vi "FL30XX.VI"() -> ()   [LabVIEW 2015]
uses:
  board.vis/Globals.vi
  board.vis/ESLSCDLL.lvlib
  board.vis/ESLSCDLL.dll
panel:
  in  "abort":bool
  in  "FFT mode":T1(ring)
  in  "is FFT":bool
  out "ADSC value":u32
  in  "Read ADSC":bool
  in  "Reset DSC":bool
  in  "CC trigger":enum32{"XCK", "Ext. Trig.", "DAT"}(ring)
  in  "STSlope":enum32{"pos", "neg", "both"}(ring)
  in  "BTSlope":enum32{"neg", "pos", "both"}(ring)=enum."pos"
  in  "btime[ms]":dbl=30.0 format="%.3f"
  out "Block on":bool
  out "String":string="with int trig:\nset exp.time accordingly\ncheck with scope!"
  in  "STI":T2(ring)=enum."STimer"
  out "TDC 2":u16
  out "TDC 1":u16
  in  "startevent":bool
  in  "BTI":enum32{"I", "S1", "S2", "S1&S2", "BTimer"}(ring)=enum."BTimer"
  in  "shutter open":bool
  in  "value black":u32
  in  "value white":u32=65535
  in  "show greyscale viewer":bool
  out "mean 3":dbl=-1.0 format="%0#.1f"
  out "tRMS 3":dbl=-1.0 format="%0#.1f"
  out "meanB":dbl=7869.371428571429 format="%0#.1f"
  out "tRMSB":dbl=13.410972192676741 format="%0#.1f"
  in  "Pixel for Graph":u32(slide)=660 max=3000 scale=0.0..1087.0
  in  "fast test\ncontinuous":bool
  out "One Pixel Graph":u16[][](graph)=[[50944, 37299, 23643, 29270, 42944, 50969, 37301, 23634, 29310, 42916, 50937, 37273, 23614, 29274, 42951, 50937, 37273, 23623, 29272, 42950, 50962, 37247, 23599, 29236, 42962, 50936, 37300, 23595, 29263, 42929, 50960, 37290, 23598, 29279, 42957, 50913, 37317, 23578, 29305, 42929, 50968, 37259, 23609, 29292, 42945, 50893, 37300, 23589, 29261, 42955, 50920, 37282, 23639, 29263, 42945, 50934, 37283, 23614, 29291, 42918, 50913, 37257, 23579, 29291, 42942, 50959, 37282, 23546, 29281, 42947, 50936, 37291, 23618, 29269, 42975, 50886, 37275, 23582, 29349, 42945, 50916, 37241, 23621, 29295, 42960, 50911, 37268, 23591, 29293, 42935, 50920, 37282, 23580, 29297, 42905, 50935, 37262, 23651, 29293, 42972, 50942, 37321, 23596, 29274, 42941, 50931, 37251, 23635, 29286, 42978, 50922, 37296, 23575, 29289, 42930, 50937, 37245, 23622, 29273, 42966, 50915, 37257, 23583, 29291, 42935, 50904, 37260, 23580, 29276, 42947, 50900, 37261, 23616, 29273, 42934, 50894, 37296, 23594, 29275, 42946, 50925, 37263, 23603, 29280, 42945, 50895, 37270, 23607, 29241, 42924, 50945, 37219, 23609, 29283, 42998, 50911, 37270, 23580, 29303, 42949, 50939, 37239, 23605, 29279, 42957, 50863, 37246, 23602, 29277, 42954, 50928, 37235, 23581, 29261, 42938, 50910, 37257, 23587, 29290, 42968, 50905, 37279, 23586, 29318, 42951, 50927, 37227, 23626, 29313, 42937, 50930, 37271, 23565, 29310, 42931, 50951, 37220, 23620, 29305, 42975, 50892, 37264, 23585, 29313, 42946, 50912, 37261, 23591, 29299, 42971, 50927, 37277, 23588, 29310, 42990, 50910, 37298, 23578, 29255, 42956, 50941, 37289, 23612, 29292, 43046, 50897, 37282, 23581, 29298, 42948, 50916, 37252, 23580, 29299, 42965, 50871, 37256, 23615, 29311, 42989, 50917, 37242, 23567, 29328, 42923, 50952, 37220, 23614, 29299, 42967, 50884, 37266, 23556, 29324, 42964, 50907, 37242, 23562, 29316, 42960, 50848, 37260, 23579, 29285, 42986, 50925, 37229, 23582, 29300, 42956, 50898, 37261, 23588, 29283, 42965, 50909, 37242, 23548, 29313, 42953, 50928, 37266, 23599, 29269, 42951, 50901, 37275, 23577, 29292, 42966, 50882, 37256, 23572, 29293, 42933, 50878, 37265, 23599, 29326, 42990, 50908, 37285, 23534, 29333, 42937, 50875, 37251, 23590, 29313, 43002, 50920, 37258, 23588, 29337, 42975, 50941, 37239, 23560, 29306, 42969, 50883, 37244, 23567, 29315, 42951, 50905, 37262, 23579, 29339, 42995, 50936, 37240, 23593, 29321, 43034, 50890, 37262, 23533, 29333, 42993, 50929, 37210, 23580, 29291, 42992, 50871, 37260, 23574, 29346, 42991, 50901, 37242, 23586, 29358, 42953, 50895, 37237, 23586, 29303, 43004, 50899, 37252, 23538, 29332, 42954, 50907, 37243, 23587, 29302, 43013, 50874, 37240, 23579, 29306, 42979, 50883, 37242, 23598, 29300, 42969, 50933, 37241, 23571, 29298, 42988, 50863, 37276, 23525, 29321, 42994, 50882, 37228, 23551, 29299, 42981, 50878, 37206, 23545, 29367, 42987, 50915, 37225, 23550, 29315, 42985, 50896, 37239, 23533, 29336, 42985, 50904, 37237, 23525, 29331, 42976, 50905, 37232, 23569, 29341, 42978, 50875, 37229, 23558, 29320, 42971, 50874, 37226, 23576, 29327, 43000, 50940, 37258, 23550, 29339, 43011, 50910, 37226, 23567, 29312, 42975, 50885, 37233, 23535, 29350, 42984, 50876, 37205, 23532, 29335, 42948, 50887, 37214, 23575, 29328, 42984, 50894, 37236, 23563, 29365, 42996, 50944, 37248, 23572, 29326, 43012, 50893, 37236, 23573, 29340, 43019, 50883, 37199, 23530, 29375, 42995, 50914, 37201, 23608, 29323, 43008, 50883, 37216, 23552, 29381, 42977, 50894, 37240, 23572, 29367, 43030, 50880, 37205, 23586, 29302, 43016, 50874, 37238, 23561, 29326, 43000]]
  in  "refresh":bool
  out "C 8":bool
  out "C 7":bool
  out "C 6":bool
  out "C 5":bool
  out "C 4":bool
  out "C 3":bool
  out "C 2":bool
  out "(LastCAM) \n        C1":bool
  out "cool_temp Reg":u32 format="%032b"
  in  "cool":u8 caption="(0 to 7)"
  in  "Offset":bool
  out "Signal Cam 4":u16[](graph)
  out "Signal Cam 3":u16[](graph)
  out "mean 2":dbl=-1.0 format="%0#.1f"
  out "meanA":dbl=33883.361224489796 format="%0#.1f"
  in  "TRMS Pix":u32=550 max=1087
  out "tRMS 2":dbl=-1.0 format="%0#.1f"
  in  "Board select":string(combo)
  in  "Initialize":bool
  in  "About S0":bool
  in  "send all":bool
  in  "DAC 8/ 1":u16=54400
  in  "DAC 3/ 1":u16=54540
  in  "DAC 7/ 1":u16=54670
  in  "DAC 2/ 1":u16=54600
  in  "DAC 6/ 1":u16=54880
  in  "DAC 1/ 1":u16=54530
  in  "DAC 5/ 1":u16=54600
  in  "DAC 4/ 1":u16=54590
  in  "custom patt: 14bits pattern hex (14bit)":u16=100 format="%x"
  out "pattern dec":fxp<+,14,14>
  in  "ADC mode":enum32{"1", "2", "3"}(radio)=enum."3"
  out "Signal Cam 2":u16[](graph)
  out "tRMSA":dbl=19568.501745308375 format="%0#.1f"
  in  "Gain":bool
  in  "framewise\ncontinuous":bool
  out "curr_read_block":u8=1
  out "Measure on":bool
  in  "no.of blocks (nob)":u32=1 min=1
  in  "block":u32(slide)=1 min=1 max=1 scale=0.9..1.0
  out "Signal Board 2 / Cam1":u16[](graph)
  out "Signal Board 1 / Cam1":u16[](graph)=[65412, 65216, 0, 1, 0, 151, 0, 0, 0, 0, 50811, 50676, 50513, 50360, 50171, 49982, 49793, 49614, 49450, 49306, 49194, 48996, 48865, 48698, 48506, 48325, 48153, 47990, 47816, 47655, 47545, 47383, 47176, 47044, 46862, 46698, 46512, 46359, 46209, 46025, 45899, 45678, 45593, 45374, 45201, 45026, 44901, 44695, 44537, 44379, 44241, 44106, 43900, 43719, 43563, 43392, 43207, 43077, 42921, 42783, 42619, 42451, 42281, 42085, 41924, 41737, 41582, 41431, 41307, 41149, 40966, 40770, 40597, 40456, 40278, 40139, 39968, 39845, 39651, 39489, 39284, 39124, 38971, 38800, 38643, 38498, 38339, 38180, 38005, 37872, 37703, 37496, 37324, 37175, 37020, 36894, 36678, 36546, 36347, 36213, 36015, 35858, 35661, 35544, 35350, 35216, 35068, 34907, 34746, 34570, 34372, 34178, 34055, 33869, 33726, 33574, 33440, 33278, 33068, 32945, 32751, 32561, 32423, 32272, 32099, 31954, 31774, 31588, 31409, 31263, 31150, 30968, 30786, 30618, 30484, 30305, 30154, 29940, 29781, 29638, 29458, 29323, 29146, 28997, 28856, 28632, 28514, 28322, 28173, 28003, 27866, 27660, 27524, 27315, 27163, 27002, 26861, 26661, 26542, 26378, 26190, 26055, 25854, 25683, 25541, 25367, 25203, 25023, 24875, 24711, 24556, 24366, 24240, 24050, 23898, 23731, 23569, 23409, 23279, 23087, 22906, 22730, 22578, 22400, 22255, 22097, 21944, 21800, 21577, 21428, 21245, 21125, 20911, 20770, 20619, 20443, 20311, 20126, 19980, 19760, 19614, 19449, 19316, 19119, 18986, 18852, 18640, 18509, 18296, 18156, 17941, 17807, 17613, 17534, 17339, 17189, 17022, 16864, 16682, 16488, 16314, 16172, 15994, 15868, 15693, 15575, 15402, 15216, 15026, 14844, 14675, 14496, 14324, 14245, 14076, 13910, 13712, 13577, 13385, 13228, 12999, 12884, 12730, 12579, 12441, 12264, 12086, 11953, 11730, 11532, 11400, 11227, 11053, 10936, 10748, 10627, 10422, 10270, 10085, 9907, 9785, 9589, 9456, 9249, 9109, 8925, 8763, 8588, 8460, 8287, 8117, 7943, 7815, 7654, 7440, 7297, 7135, 6957, 6789, 6631, 6490, 6301, 6139, 5965, 5813, 5661, 5492, 5342, 5212, 4985, 4872, 4637, 4441, 4306, 4206, 4013, 3889, 3690, 3542, 3385, 3189, 3025, 2874, 2709, 2513, 2368, 2205, 2056, 1910, 1719, 1555, 1402, 1212, 1082, 907, 752, 605, 445, 258, 72, 0, 0, 0, 0, 0, 0, 0, 0, 0, 0, 0, 0, 151, 312, 511, 714, 849, 1024, 1166, 1300, 1482, 1649, 1819, 2010, 2112, 2346, 2468, 2649, 2803, 2967, 3134, 3309, 3503, 3626, 3822, 3902, 4115, 4247, 4442, 4599, 4750, 4965, 5102, 5270, 5376, 5612, 5729, 5904, 6071, 6270, 6459, 6598, 6780, 6883, 7065, 7226, 7356, 7543, 7760, 7915, 8075, 8235, 8382, 8518, 8701, 8868, 9028, 9228, 9389, 9560, 9740, 9861, 10039, 10193, 10345, 10490, 10703, 10875, 11058, 11215, 11376, 11527, 11658, 11832, 11992, 12171, 12336, 12545, 12706, 12875, 13023, 13161, 13315, 13483, 13636, 13778, 14006, 14173, 14347, 14464, 14689, 14809, 14997, 15163, 15301, 15499, 15644, 15844, 15961, 16116, 16283, 16443, 16623, 16806, 16971, 17146, 17333, 17437, 17646, 17763, 17935, 18076, 18241, 18408, 18591, 18758, 18897, 19096, 19258, 19440, 19564, 19754, 19895, 20074, 20212, 20376, 20542, 20753, 20884, 21097, 21209, 21412, 21546, 21692, 21879, 22022, 22223, 22345, 22551, 22715, 22894, 23017, 23193, 23325, 23485, 23694, 23841, 23987, 24201, 24357, 24522, 24691, 24825, 24954, 25106, 25283, 25468, 25683, 25862, 26023, 26162, 26287, 26450, 26604, 26776, 26941, 27150, 27306, 27475, 27649, 27799, 27935, 28099, 28219, 28422, 28589, 28811, 28965, 29145, 29250, 29438, 29573, 29718, 29898, 30077, 30229, 30440, 30612, 30759, 30921, 31056, 31211, 31363, 31533, 31712, 31879, 32067, 32239, 32414, 32534, 32696, 32850, 33030, 33204, 33360, 33537, 33724, 33842, 34021, 34178, 34329, 34488, 34642, 34835, 35007, 35191, 35336, 35497, 35663, 35816, 35973, 36131, 36313, 36476, 36625, 36803, 36950, 37174, 37281, 37426, 37646, 37801, 37959, 38128, 38270, 38460, 38603, 38746, 38931, 39098, 39240, 39453, 39608, 39758, 39913, 40107, 40240, 40411, 40603, 40736, 40910, 41078, 41218, 41421, 41540, 41722, 41844, 42060, 42227, 42437, 42539, 42747, 42860, 43039, 43169, 43356, 43493, 43688, 43818, 44024, 44220, 44357, 44504, 44666, 44818, 44990, 45166, 45331, 45498, 45656, 45806, 45964, 46151, 46312, 46469, 46655, 46820, 46956, 47139, 47276, 47489, 47620, 47774, 47975, 48121, 48294, 48468, 48599, 48782, 48923, 49091, 49240, 49408, 49596, 49777, 49943, 50096, 50263, 50415, 50577, 50740, 50910, 51082, 51247, 51421, 51570, 51778, 51885, 52034, 52181, 52353, 52531, 52735, 52898, 53058, 53223, 53371, 53516, 53666, 53826, 54005, 54205, 54349, 54512, 54736, 54859, 55012, 55161, 55342, 55492, 55645, 55844, 56018, 56186, 56352, 56502, 56656, 56808, 56958, 57179, 57337, 57518, 57656, 57795, 57962, 58123, 58277, 58458, 58625, 58804, 58966, 59150, 59290, 59459, 59580, 59791, 59941, 60088, 60291, 60460, 60650, 60812, 60923, 61089, 61240, 61405, 61541, 61790, 61941, 62115, 62312, 62444, 62600, 62748, 62871, 63033, 63232, 63414, 63536, 63763, 63880, 64071, 64261, 64380, 64539, 64683, 64825, 65040, 65200, 65394, 65535, 65535, 65535, 65535, 65535, 65535, 65535, 65535, 65535, 65535, 65535, 65535, 65535, 65535, 65535, 65535, 65535, 65535, 65535, 65535, 65535, 65535, 65535, 65535, 65524, 65296, 65146, 64951, 64825, 64641, 64532, 64393, 64226, 64044, 63834, 63698, 63474, 63328, 63164, 63032, 62887, 62732, 62570, 62386, 62221, 62017, 61833, 61682, 61546, 61383, 61215, 61054, 60948, 60729, 60571, 60359, 60199, 60035, 59886, 59745, 59581, 59449, 59265, 59104, 58921, 58730, 58519, 58380, 58244, 58091, 57962, 57834, 57638, 57364, 57279, 57079, 56920, 56742, 56603, 56469, 56296, 56154, 55934, 55788, 55584, 55418, 55262, 55114, 54960, 54795, 54678, 54443, 54307, 54139, 53955, 53792, 53623, 53469, 53299, 53172, 53022, 52830, 52666, 52490, 52310, 52166, 51986, 51857, 51662, 51548, 51342, 51181, 51000, 50837, 50660, 50492, 50391, 50188, 50085, 49874, 49714, 49544, 49353, 49160, 49039, 48877, 48737, 48557, 48401, 48225, 48041, 47935, 47725, 47585, 47401, 47231, 47125, 46913, 46782, 46573, 46416, 46223, 46071, 45886, 45758, 45614, 45445, 45276, 45122, 44964, 44782, 44608, 44424, 44220, 44103, 43949, 43789, 43649, 43479, 43305, 43148, 42969, 42834, 42621, 42507, 42316, 42140, 41985, 41838, 41659, 41486, 41342, 41163, 41025, 40849, 40651, 40502, 40364, 40171, 40025, 39852, 39696, 39497, 39388, 39188, 39029, 38880, 38701, 38568, 38414, 38214, 38081, 37855, 37727, 37486, 37388, 37210, 37080, 36908, 36768, 36606, 36395, 36247, 36093, 35904, 35738, 35582, 35420, 35274, 35111, 34923, 34765, 34602, 34448, 34314, 34120, 33941, 33814, 33596, 33493, 33276, 33132, 32966, 32821, 32630, 32501, 32322, 32144, 31968, 31816, 31667, 31515, 31347, 31183, 31019, 30860, 30678, 30521, 30333, 30179, 30001, 29870, 29707, 29566, 29413, 29221, 29032, 28817, 28696, 28474, 28364, 28217, 28054, 27918, 27741, 27575, 27401, 27211, 27035, 26852, 26699, 26562, 26404, 26274, 26125, 25942, 25754, 25563, 25405, 25223, 25082, 24938, 24794, 24628, 24465, 24277, 24152, 23901, 23772, 23583, 23462, 23288, 23165, 22985, 22829, 22650, 22457, 22302, 22085, 21979, 21818, 21652, 21537, 21331, 21172, 20948, 20846, 20664, 20477, 20358, 20181, 20033, 19847, 19702, 19524, 19360, 19171, 19025, 18836, 18707, 18533, 18375, 18219, 18066, 17894, 17716, 17586, 17348, 17195, 17043, 16880, 16746, 16540, 16414, 16226, 16086, 15916, 15761, 15567, 15436, 15228, 15083, 14916, 14783, 14582, 14447, 14259, 14103, 13948, 13777, 13612, 13443, 13285, 13106, 12993, 12807, 12591, 12454, 12268, 12125, 11948, 11817, 65534, 65535, 0, 0, 2, 0]
  out "# boards \ndetected":u32=1
  in  "alloc mem":bool
  out "FREE \nRAM MB":dbl=29213.2109375
  out "BUILT-IN\nRAM MB":dbl=32640.29296875
  out "SEC":dbl=0.1
  out "MB RAM":dbl=1.03759765625
  in  "SDAT in 10ns":u32
  in  "exit":bool
  in  "start":bool
  in  "sample":u32(slide)=151 min=1 max=20 scale=1.0..20.0
  in  "no.of samples (nos)":u32=20 min=2
  in  "stime[ms]":dbl=1.0 format="%.3f"
  # "press \"Initialize\", then \"alloc mem\"\nand then \"start\""
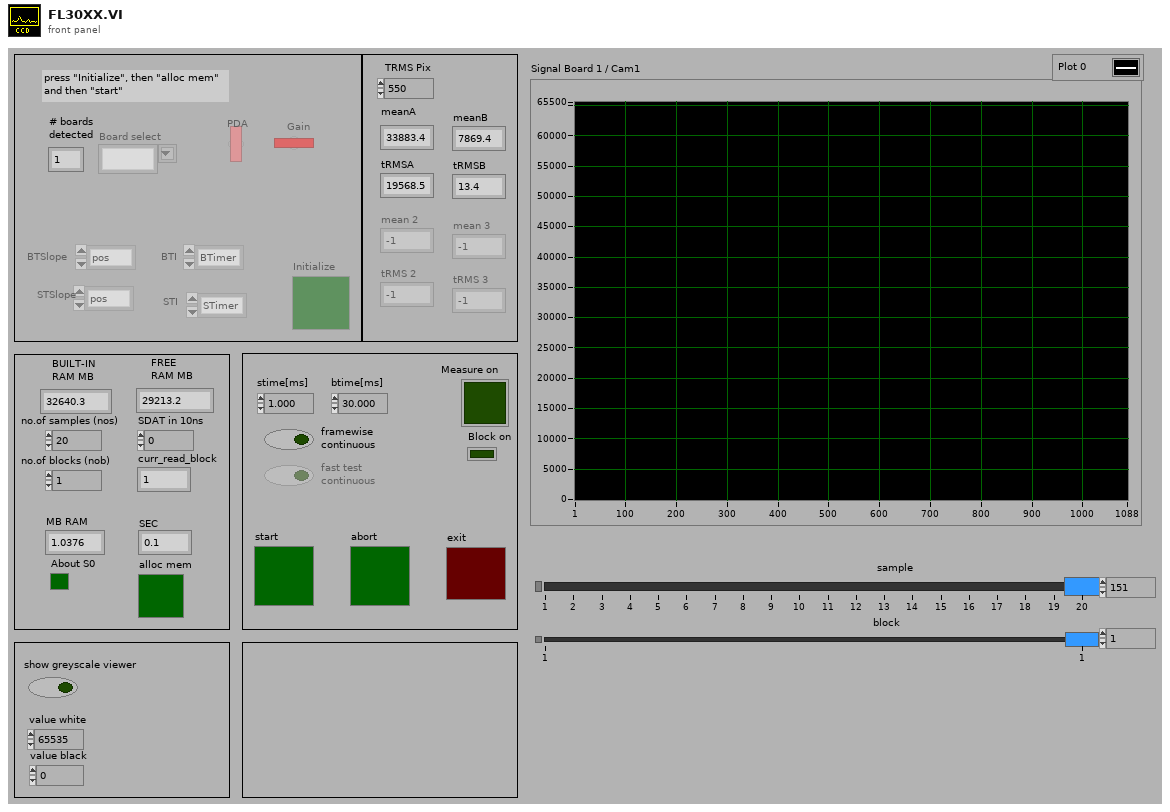
[diagram p1: front panel]
types:
  T1 = enum32{"Full Binning", "Region of Interest", "Area"}
  T2 = enum32{"I", "S1", "S2", "unused", "STimer", "ASL"}
  T3 = enum32{"XCK", "Reg/OutTrig", "VON", "DMA_Act", "ASLS", "STIMER", "BTIMER", "INTRSR", "S1", "S2", "BON", "MEASUREON", "SDAT", "BDAT", "SSHUT", "BSHUT"}
  T4 = enum8{"Enabled", "Disabled", "Disabled and Grayed Out"}
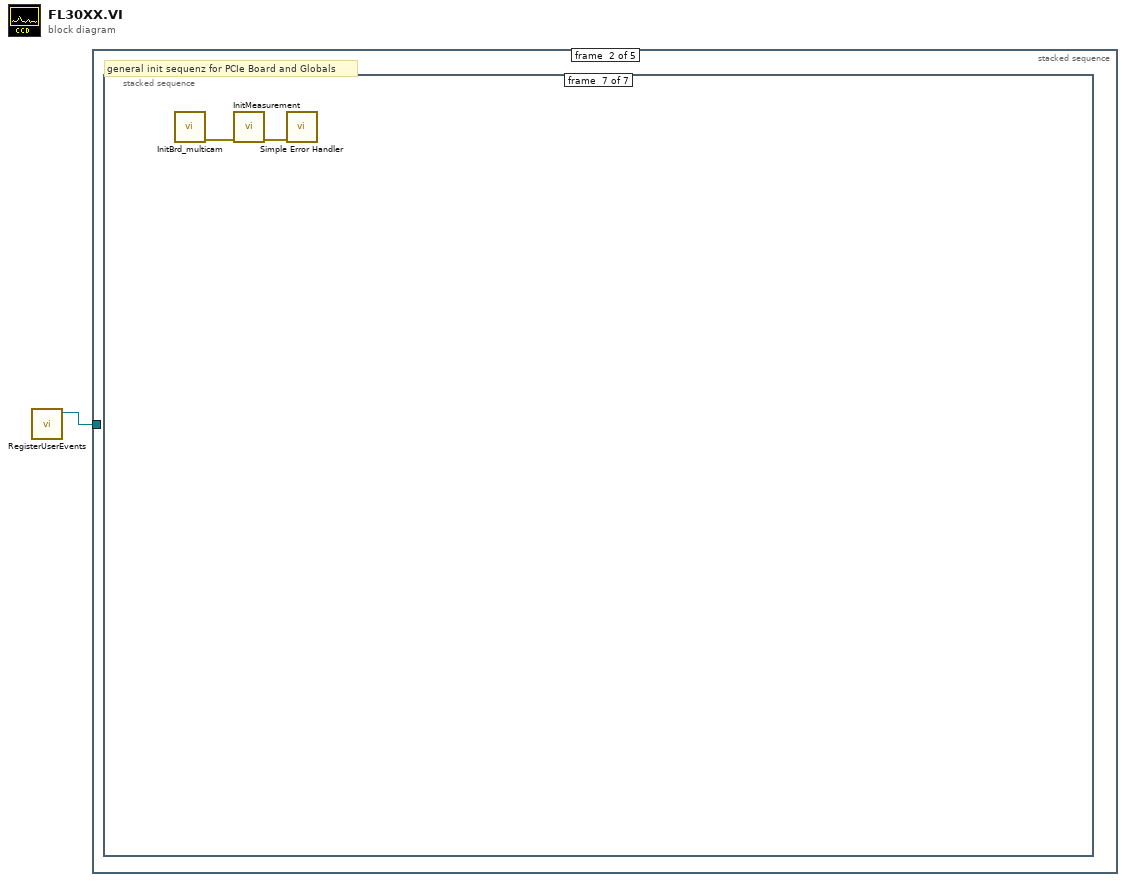
[diagram p0: block diagram]
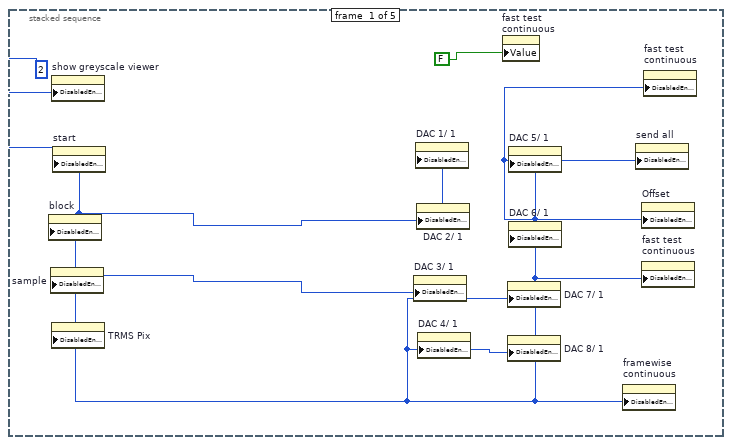
[diagram p2: hidden frame]
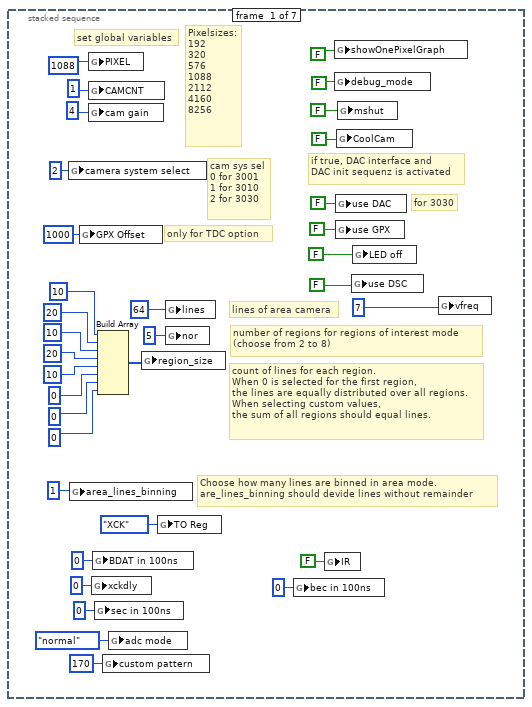
[diagram p3: hidden frame]
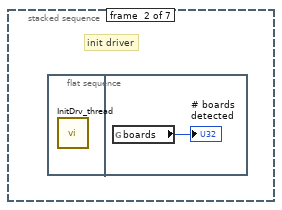
[diagram p4: hidden frame]
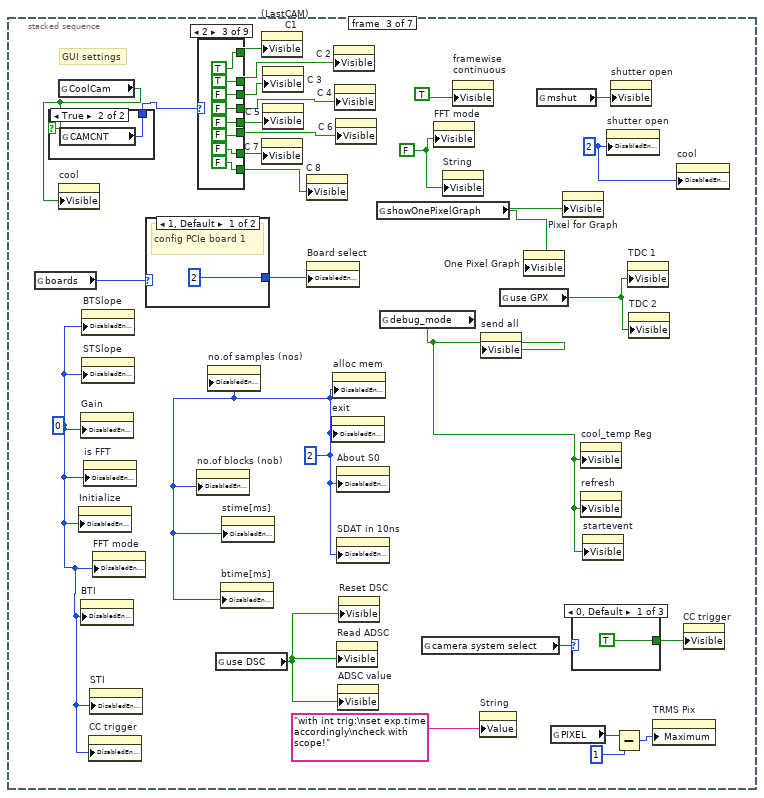
[diagram p5: hidden frame]
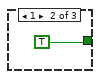
[diagram p6: hidden frame]
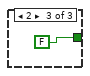
[diagram p7: hidden frame]
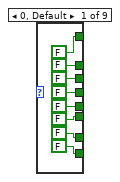
[diagram p8: hidden frame]
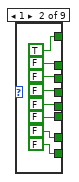
[diagram p9: hidden frame]
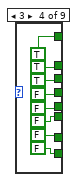
[diagram p10: hidden frame]
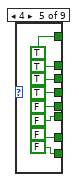
[diagram p11: hidden frame]
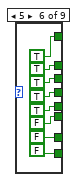
[diagram p12: hidden frame]
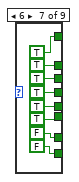
[diagram p13: hidden frame]
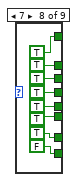
[diagram p14: hidden frame]
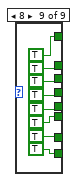
[diagram p15: hidden frame]
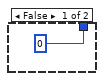
[diagram p16: hidden frame]
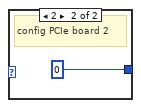
[diagram p17: hidden frame]
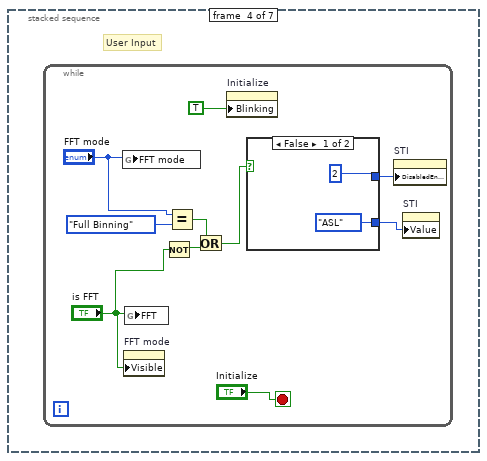
[diagram p18: hidden frame]
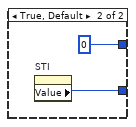
[diagram p19: hidden frame]
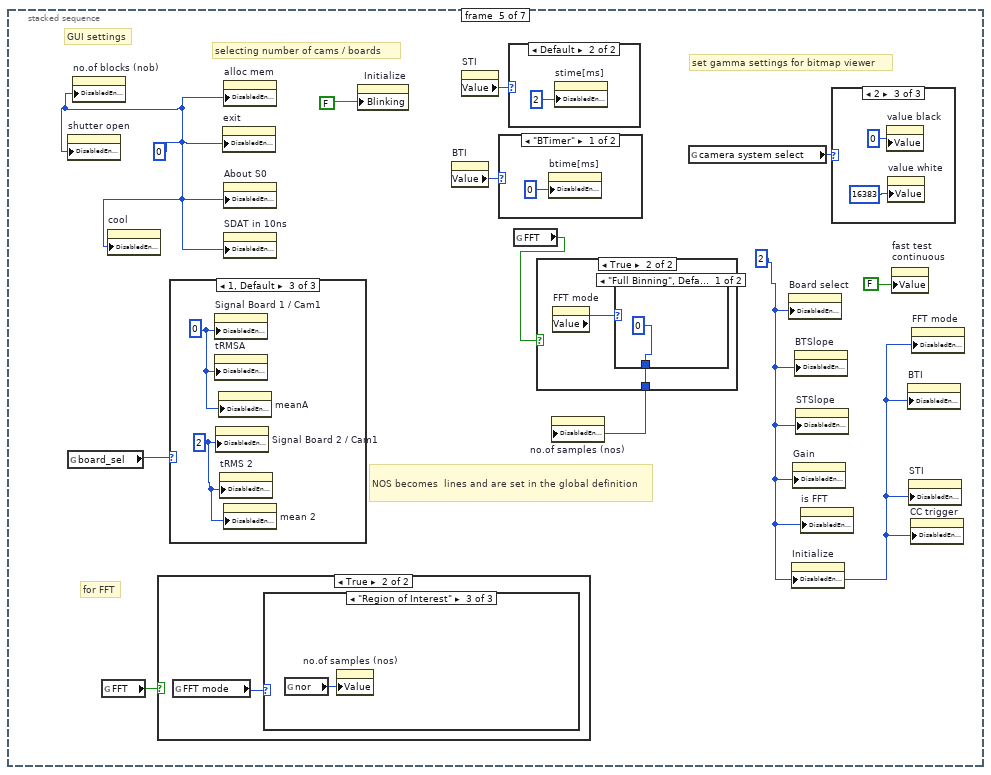
[diagram p20: hidden frame]
diagram:
  n1 = call "RegisterUserEvents.vi"() -> ("Event Registration Refnum"=w1:refnum<event-registration>)  [unwired: 10 in, 1 out]
  n2 = stacked-sequence {
    tunnel: w1 -> [_ _ _ _ w280]
    frame #0 {
      w2 = 2
      n3 = property on="block" class="Slide (strict)"("DisabledEnum"=w2) -> ()  [unwired: 2 in, 2 out]
      n4 = property on="sample" class="Slide (strict)"("DisabledEnum"=w2) -> ()  [unwired: 2 in, 2 out]
      n5 = property on="show greyscale viewer" class="Bool (strict)"("DisabledEnum"=w2) -> ()  [unwired: 2 in, 2 out]
      n6 = property on="TRMS Pix" class="DigNum (strict)"("DisabledEnum"=w2) -> ()  [unwired: 2 in, 2 out]
      n7 = property on="start" class="Bool (strict)"("DisabledEnum"=w2) -> ()  [unwired: 2 in, 2 out]
      n8 = property on="DAC 3/ 1" class="DigNum (strict)"("DisabledEnum"=w2) -> ()  [unwired: 2 in, 2 out]
      n9 = property on="DAC 1/ 1" class="DigNum (strict)"("DisabledEnum"=w2) -> ()  [unwired: 2 in, 2 out]
      n10 = property on="DAC 2/ 1" class="DigNum (strict)"("DisabledEnum"=w2) -> ()  [unwired: 2 in, 2 out]
      n11 = property on="DAC 4/ 1" class="DigNum (strict)"("DisabledEnum"=w2) -> ()  [unwired: 2 in, 2 out]
      n12 = property on="fast test\ncontinuous" class="Bool (strict)"("Value"=FALSE) -> ()  [unwired: 2 in, 2 out]
      n13 = property on="DAC 7/ 1" class="DigNum (strict)"("DisabledEnum"=w2) -> ()  [unwired: 2 in, 2 out]
      n14 = property on="DAC 8/ 1" class="DigNum (strict)"("DisabledEnum"=w2) -> ()  [unwired: 2 in, 2 out]
      n15 = property on="DAC 5/ 1" class="DigNum (strict)"("DisabledEnum"=w2) -> ()  [unwired: 2 in, 2 out]
      n16 = property on="DAC 6/ 1" class="DigNum (strict)"("DisabledEnum"=w2) -> ()  [unwired: 2 in, 2 out]
      n17 = property on="framewise\ncontinuous" class="Bool (strict)"("DisabledEnum"=w2) -> ()  [unwired: 2 in, 2 out]
      n18 = property on="send all" class="Bool (strict)"("DisabledEnum"=w2) -> ()  [unwired: 2 in, 2 out]
      n19 = property on="Offset" class="Bool (strict)"("DisabledEnum"=w2) -> ()  [unwired: 2 in, 2 out]
      n20 = property on="fast test\ncontinuous" class="Bool (strict)"("DisabledEnum"=w2) -> ()  [unwired: 2 in, 2 out]
      n21 = property on="fast test\ncontinuous" class="Bool (strict)"("DisabledEnum"=w2) -> ()  [unwired: 2 in, 2 out]
    }
    frame #1 {
      # "general init sequenz for PCIe Board and Globals"
      n22 = stacked-sequence {
        frame #0 {
          # "Choose how many lines are binned in area mode.\nare_lines_binning should devide lines without remainder"
          # "count of lines for each region.\nWhen 0 is selected for the first region,\nthe lines are equally distributed over all regions.\nWhen selecting custom values,\nthe sum of all regions should equal lines."
          # "number of regions for regions of interest mode\n(choose from 2 to 8)"
          # "lines of area camera"
          # "only for TDC option"
          # "Pixelsizes:\n192\n320\n576\n1088\n2112\n4160\n8256"
          # "if true, DAC interface and \nDAC init sequenz is activated"
          # "for 3030"
          # "set global variables"
          # "cam sys sel\n0 for 3001\n1 for 3010\n2 for 3030"
          n23 = global write "Globals.vi" "camera system select"(u32 2) -> ()
          n24 = global write "Globals.vi" "area_lines_binning"(u32 1) -> ()
          n25 = global write "Globals.vi" "GPX Offset"(u32 1000) -> ()
          n26 = global write "Globals.vi" "PIXEL"(u32 1088) -> ()
          n27 = global write "Globals.vi" "CAMCNT"(u32 1) -> ()
          n28 = global write "Globals.vi" "cam gain"(u32 4) -> ()
          n29 = global write "Globals.vi" "xckdly"(u32 0 ("xckdly")) -> ()
          n30 = global write "Globals.vi" "BDAT in 100ns"(u32 0 ("BDAT in 100ns")) -> ()
          n31 = global write "Globals.vi" "sec in 100ns"(u32 0 ("sec in 100ns")) -> ()
          n32 = Build Array(u32 10, u32 20, u32 10, u32 20, u32 10, u32 0, u32 0, u32 0) -> (w16:u32[])
          n33 = global write "Globals.vi" "custom pattern"(u32 170 ("custom pattern")) -> ()
          n34 = global write "Globals.vi" "adc mode"(enum16{"normal", "ramp", "custom pattern"}."normal" ("adc mode")) -> ()
          n35 = global write "Globals.vi" "region_size"(w16) -> ()
          n36 = global write "Globals.vi" "TO Reg"(T3."XCK" ("TO Reg")) -> ()
          n37 = global write "Globals.vi" "lines"(u32 64) -> ()
          n38 = global write "Globals.vi" "nor"(u32 5) -> ()
          n39 = global write "Globals.vi" "bec in 100ns"(u32 0 ("bec in 100ns")) -> ()
          n40 = global write "Globals.vi" "IR"(FALSE ("IR")) -> ()
          n41 = global write "Globals.vi" "showOnePixelGraph"(FALSE) -> ()
          n42 = global write "Globals.vi" "debug_mode"(FALSE) -> ()
          n43 = global write "Globals.vi" "use DAC"(FALSE) -> ()
          n44 = global write "Globals.vi" "use GPX"(FALSE) -> ()
          n45 = global write "Globals.vi" "CoolCam"(FALSE) -> ()
          n46 = global write "Globals.vi" "mshut"(FALSE) -> ()
          n47 = global write "Globals.vi" "use DSC"(FALSE) -> ()
          n48 = global write "Globals.vi" "LED off"(FALSE) -> ()
          n49 = global write "Globals.vi" "vfreq"(u32 7) -> ()
        }
        frame #1 {
          # "init driver"
          n50 = flat-sequence {
            frame #0 {
              n51 = call "InitDrv_thread.vi"() -> ()  [unwired: 11 in, 1 out]
            }
            frame #1 {
              n52 = global read "Globals.vi" "boards"() -> (→"# boards \ndetected":u32)
            }
          }
        }
        frame #2 {
          w39 = 2
          w41 = FALSE
          w40 = 0
          w48 = 2
          # "GUI settings"
          n53 = global read "Globals.vi" "boards"() -> (w65:u32)
          n54 = global read "Globals.vi" "CoolCam"() -> (w54:bool)
          n55 = case shown="True" w54 {
            tunnel: [u32 0 w143] -> w63
            frame False {
            }
            frame True {
              n56 = global read "Globals.vi" "CAMCNT"() -> (w143:u32)
            }
          }
          n57 = property on="cool" class="DigNum (strict)"("Visible"=w54) -> ()  [unwired: 2 in, 2 out]
          n58 = property on="Initialize" class="Bool (strict)"("DisabledEnum"=w40) -> ()  [unwired: 2 in, 2 out]
          n59 = property on="Gain" class="Bool (strict)"("DisabledEnum"=w40) -> ()  [unwired: 2 in, 2 out]
          n60 = property on="BTI" class="Enum (strict)"("DisabledEnum"=w40) -> ()  [unwired: 2 in, 2 out]
          n61 = property on="BTSlope" class="Enum (strict)"("DisabledEnum"=w40) -> ()  [unwired: 2 in, 2 out]
          n62 = property on="STSlope" class="Enum (strict)"("DisabledEnum"=w40) -> ()  [unwired: 2 in, 2 out]
          n63 = property on="is FFT" class="Bool (strict)"("DisabledEnum"=w40) -> ()  [unwired: 2 in, 2 out]
          n64 = property on="CC trigger" class="Enum (strict)"("DisabledEnum"=w40) -> ()  [unwired: 2 in, 2 out]
          n65 = property on="STI" class="Enum (strict)"("DisabledEnum"=w40) -> ()  [unwired: 2 in, 2 out]
          n66 = property on="FFT mode" class="Enum (strict)"("DisabledEnum"=w40) -> ()  [unwired: 2 in, 2 out]
          n67 = case shown="1, Default" w65 {
            tunnel: [2 0] -> w66
            frame 1, Default {
              # "config PCIe board 1"
            }
            frame 2 {
              # "config PCIe board 2"
            }
          }
          n68 = property on="no.of blocks (nob)" class="DigNum (strict)"("DisabledEnum"=w48) -> ()  [unwired: 2 in, 2 out]
          n69 = case shown="2" w63 {
            tunnel: [FALSE TRUE TRUE TRUE TRUE TRUE TRUE TRUE TRUE] -> w62
            tunnel: [FALSE FALSE FALSE TRUE TRUE TRUE TRUE TRUE TRUE] -> w61
            tunnel: [FALSE FALSE FALSE FALSE TRUE TRUE TRUE TRUE TRUE] -> w60
            tunnel: [FALSE FALSE FALSE FALSE FALSE TRUE TRUE TRUE TRUE] -> w59
            tunnel: [FALSE FALSE FALSE FALSE FALSE FALSE TRUE TRUE TRUE] -> w58
            tunnel: [FALSE FALSE FALSE FALSE FALSE FALSE FALSE TRUE TRUE] -> w57
            tunnel: [FALSE FALSE FALSE FALSE FALSE FALSE FALSE FALSE TRUE] -> w56
            tunnel: [FALSE FALSE TRUE TRUE TRUE TRUE TRUE TRUE TRUE] -> w55
            frame 0, Default {
            }
            frame 1 {
            }
            frame 2 {
            }
            frame 3 {
            }
            frame 4 {
            }
            frame 5 {
            }
            frame 6 {
            }
            frame 7 {
            }
            frame 8 {
            }
          }
          n70 = property on="no.of samples (nos)" class="DigNum (strict)"("DisabledEnum"=w48) -> ()  [unwired: 2 in, 2 out]
          n71 = global read "Globals.vi" "use DSC"() -> (w45:bool)
          n72 = property on="btime[ms]" class="DigNum (strict)"("DisabledEnum"=w48) -> ()  [unwired: 2 in, 2 out]
          n73 = property on="stime[ms]" class="DigNum (strict)"("DisabledEnum"=w48) -> ()  [unwired: 2 in, 2 out]
          n74 = property on="(LastCAM) \n        C1" class="Bool (strict)"("Visible"=w62) -> ()  [unwired: 2 in, 2 out]
          n75 = property on="C 7" class="Bool (strict)"("Visible"=w57) -> ()  [unwired: 2 in, 2 out]
          n76 = property on="C 3" class="Bool (strict)"("Visible"=w61) -> ()  [unwired: 2 in, 2 out]
          n77 = property on="C 5" class="Bool (strict)"("Visible"=w59) -> ()  [unwired: 2 in, 2 out]
          n78 = property on="C 8" class="Bool (strict)"("Visible"=w56) -> ()  [unwired: 2 in, 2 out]
          n79 = property on="Board select" class="CmbBox"("DisabledEnum"=w66) -> ()  [unwired: 2 in, 2 out]
          n80 = property on="exit" class="Bool (strict)"("DisabledEnum"=w48) -> ()  [unwired: 2 in, 2 out]
          n81 = property on="alloc mem" class="Bool (strict)"("DisabledEnum"=w48) -> ()  [unwired: 2 in, 2 out]
          n82 = property on="C 2" class="Bool (strict)"("Visible"=w55) -> ()  [unwired: 2 in, 2 out]
          n83 = property on="C 4" class="Bool (strict)"("Visible"=w60) -> ()  [unwired: 2 in, 2 out]
          n84 = property on="C 6" class="Bool (strict)"("Visible"=w58) -> ()  [unwired: 2 in, 2 out]
          n85 = property on="About S0" class="Bool (strict)"("DisabledEnum"=w48) -> ()  [unwired: 2 in, 2 out]
          n86 = property on="SDAT in 10ns" class="DigNum (strict)"("DisabledEnum"=w48) -> ()  [unwired: 2 in, 2 out]
          n87 = property on="Read ADSC" class="Bool (strict)"("Visible"=w45) -> ()  [unwired: 2 in, 2 out]
          n88 = property on="ADSC value" class="DigNum (strict)"("Visible"=w45) -> ()  [unwired: 2 in, 2 out]
          n89 = property on="Reset DSC" class="Bool (strict)"("Visible"=w45) -> ()  [unwired: 2 in, 2 out]
          n90 = global read "Globals.vi" "showOnePixelGraph"() -> (w53:bool)
          n91 = global read "Globals.vi" "debug_mode"() -> (w51:bool)
          n92 = global read "Globals.vi" "camera system select"() -> (w47:u32)
          n93 = property on="FFT mode" class="Enum (strict)"("Visible"=w41) -> ()  [unwired: 2 in, 2 out]
          n94 = property on="String" class="Str"("Visible"=w41) -> ()  [unwired: 2 in, 2 out]
          n95 = property on="framewise\ncontinuous" class="Bool (strict)"("Visible"=TRUE) -> ()  [unwired: 2 in, 2 out]
          n96 = property on="String" class="Str"("Value"="with int trig:\nset exp.time accordingly\ncheck with scope!") -> ()  [unwired: 2 in, 2 out]
          n97 = property on="send all" class="Bool (strict)"("Visible"=w51) -> ()  [unwired: 2 in, 2 out]
          n98 = global read "Globals.vi" "use GPX"() -> (w50:bool)
          n99 = property on="One Pixel Graph" class="WFGraph (strict)"("Visible"=w53) -> ()  [unwired: 2 in, 2 out]
          n100 = global read "Globals.vi" "mshut"() -> (w52:bool)
          n101 = global read "Globals.vi" "PIXEL"() -> (w44:u32)
          n102 = property on="Pixel for Graph" class="Slide (strict)"("Visible"=w53) -> ()  [unwired: 2 in, 2 out]
          n103 = case shown="0, Default" w47 {
            tunnel: [TRUE TRUE FALSE] -> w46
            frame 0, Default {
            }
            frame 1 {
            }
            frame 2 {
            }
          }
          n104 = property on="cool_temp Reg" class="DigNum (strict)"("Visible"=w51) -> ()  [unwired: 2 in, 2 out]
          n105 = property on="refresh" class="Bool (strict)"("Visible"=w51) -> ()  [unwired: 2 in, 2 out]
          n106 = property on="startevent" class="Bool (strict)"("Visible"=w51) -> ()  [unwired: 2 in, 2 out]
          n107 = property on="shutter open" class="Bool (strict)"("DisabledEnum"=w39) -> ()  [unwired: 2 in, 2 out]
          n108 = property on="shutter open" class="Bool (strict)"("Visible"=w52) -> ()  [unwired: 2 in, 2 out]
          n109 = Subtract(x=w44, y=u32 1) -> (x-y=w43:u32)
          n110 = property on="TDC 1" class="DigNum (strict)"("Visible"=w50) -> ()  [unwired: 2 in, 2 out]
          n111 = property on="TDC 2" class="DigNum (strict)"("Visible"=w50) -> ()  [unwired: 2 in, 2 out]
          n112 = property on="TRMS Pix" class="DigNum (strict)"("Maximum"=w43) -> ()  [unwired: 2 in, 2 out]
          n113 = property on="cool" class="DigNum (strict)"("DisabledEnum"=w39) -> ()  [unwired: 2 in, 2 out]
          n114 = property on="CC trigger" class="Enum (strict)"("Visible"=w46) -> ()  [unwired: 2 in, 2 out]
        }
        frame #3 {
          # "User Input"
          n115 = while {
            stop <- "Initialize" stop-if-true
            n116 = global write "Globals.vi" "FFT mode"("FFT mode") -> ()
            n117 = property on="FFT mode" class="Enum (strict)"("Visible"="is FFT") -> ()  [unwired: 2 in, 2 out]
            n118 = global write "Globals.vi" "FFT"("is FFT") -> ()
            n119 = Not(x="is FFT") -> (.not. x?=w150:bool)
            n120 = Equal?(x="FFT mode", y=T1."Full Binning") -> (x = y?=w148:bool)
            n121 = Or(x=w148, y=w150) -> (x .or. y?=w151:bool)
            n122 = property on="Initialize" class="Bool (strict)"("Blinking"=TRUE) -> ()  [unwired: 2 in, 2 out]
            n123 = case shown="False" w151 {
              tunnel: [2 0] -> w153
              tunnel: [T2."ASL" ("Value") w158] -> w152
              frame False {
              }
              frame True, Default {
                n124 = property on="STI" class="Enum (strict)"() -> ("Value"=w158:T2)  [unwired: 2 in, 2 out]
              }
            }
            n125 = property on="STI" class="Enum (strict)"("DisabledEnum"=w153) -> ()  [unwired: 2 in, 2 out]
            n126 = property on="STI" class="Enum (strict)"("Value"=w152) -> ()  [unwired: 2 in, 2 out]
          }
        }
        frame #4 {
          w163 = u8 2
          w160 = i8 0
          # "for FFT"
          # "set gamma settings for bitmap viewer"
          # "NOS becomes  lines and are set in the global definition"
          # "GUI settings"
          # "selecting number of cams / boards"
          n127 = property on="shutter open" class="Bool (strict)"("DisabledEnum"=w160) -> ()  [unwired: 2 in, 2 out]
          n128 = global read "Globals.vi" "board_sel"() -> (w169:u32)
          n129 = property on="no.of blocks (nob)" class="DigNum (strict)"("DisabledEnum"=w160) -> ()  [unwired: 2 in, 2 out]
          n130 = global read "Globals.vi" "FFT"() -> (w161:bool)
          n131 = property on="cool" class="DigNum (strict)"("DisabledEnum"=w160) -> ()  [unwired: 2 in, 2 out]
          n132 = case shown="True" w161 {
            frame False {
              # "turn partial binning off"
            }
            frame True {
              n133 = global read "Globals.vi" "FFT mode"() -> (w171:T1)
              n134 = case shown="\"Region of Interest\"" w171 {
                frame "Full Binning", Default {
                }
                frame "Area" {
                  # "set to ASL"
                  n135 = global read "Globals.vi" "area_lines_binning"() -> (w174:u32)
                  n136 = global read "Globals.vi" "lines"() -> (w175:u32)
                  n137 = Divide(x=w175, y=w174) -> (x/y=w172:dbl)
                  n138 = To Unsigned Long Integer(number=w172) -> (unsigned 32bit integer=w173:u32)
                  n139 = property on="no.of samples (nos)" class="DigNum (strict)"("Value"=w173) -> ()  [unwired: 2 in, 2 out]
                }
                frame "Region of Interest" {
                  n140 = global read "Globals.vi" "nor"() -> (w176:u32)
                  n141 = property on="no.of samples (nos)" class="DigNum (strict)"("Value"=w176) -> ()  [unwired: 2 in, 2 out]
                }
              }
            }
          }
          n142 = case shown="1, Default" w169 {
            frame 2 {
              w192 = 0
              w193 = 2
              n143 = property on="Signal Board 1 / Cam1" class="WFGraph (strict)"("DisabledEnum"=w193) -> ()  [unwired: 2 in, 2 out]
              n144 = property on="tRMSA" class="DigNum (strict)"("DisabledEnum"=w193) -> ()  [unwired: 2 in, 2 out]
              n145 = property on="Signal Board 2 / Cam1" class="WFGraph (strict)"("DisabledEnum"=w192) -> ()  [unwired: 2 in, 2 out]
              n146 = property on="meanA" class="DigNum (strict)"("DisabledEnum"=w193) -> ()  [unwired: 2 in, 2 out]
              n147 = property on="tRMS 2" class="DigNum (strict)"("DisabledEnum"=w192) -> ()  [unwired: 2 in, 2 out]
              n148 = property on="mean 2" class="DigNum (strict)"("DisabledEnum"=w192) -> ()  [unwired: 2 in, 2 out]
            }
            frame 3 {
              w194 = 0
              w195 = 0
              n149 = property on="Signal Board 1 / Cam1" class="WFGraph (strict)"("DisabledEnum"=w195) -> ()  [unwired: 2 in, 2 out]
              n150 = property on="tRMSA" class="DigNum (strict)"("DisabledEnum"=w195) -> ()  [unwired: 2 in, 2 out]
              n151 = property on="Signal Board 2 / Cam1" class="WFGraph (strict)"("DisabledEnum"=w194) -> ()  [unwired: 2 in, 2 out]
              n152 = property on="meanA" class="DigNum (strict)"("DisabledEnum"=w195) -> ()  [unwired: 2 in, 2 out]
              n153 = property on="tRMS 2" class="DigNum (strict)"("DisabledEnum"=w194) -> ()  [unwired: 2 in, 2 out]
              n154 = property on="mean 2" class="DigNum (strict)"("DisabledEnum"=w194) -> ()  [unwired: 2 in, 2 out]
            }
            frame 1, Default {
              w196 = 2
              w197 = 0
              n155 = property on="Signal Board 1 / Cam1" class="WFGraph (strict)"("DisabledEnum"=w197) -> ()  [unwired: 2 in, 2 out]
              n156 = property on="tRMSA" class="DigNum (strict)"("DisabledEnum"=w197) -> ()  [unwired: 2 in, 2 out]
              n157 = property on="Signal Board 2 / Cam1" class="WFGraph (strict)"("DisabledEnum"=w196) -> ()  [unwired: 2 in, 2 out]
              n158 = property on="meanA" class="DigNum (strict)"("DisabledEnum"=w197) -> ()  [unwired: 2 in, 2 out]
              n159 = property on="tRMS 2" class="DigNum (strict)"("DisabledEnum"=w196) -> ()  [unwired: 2 in, 2 out]
              n160 = property on="mean 2" class="DigNum (strict)"("DisabledEnum"=w196) -> ()  [unwired: 2 in, 2 out]
            }
          }
          n161 = property on="exit" class="Bool (strict)"("DisabledEnum"=w160) -> ()  [unwired: 2 in, 2 out]
          n162 = property on="alloc mem" class="Bool (strict)"("DisabledEnum"=w160) -> ()  [unwired: 2 in, 2 out]
          n163 = property on="About S0" class="Bool (strict)"("DisabledEnum"=w160) -> ()  [unwired: 2 in, 2 out]
          n164 = property on="SDAT in 10ns" class="DigNum (strict)"("DisabledEnum"=w160) -> ()  [unwired: 2 in, 2 out]
          n165 = property on="Initialize" class="Bool (strict)"("Blinking"=FALSE) -> ()  [unwired: 2 in, 2 out]
          n166 = property on="BTI" class="Enum (strict)"() -> ("Value"=w165:enum32{"I", "S1", "S2", "S1&S2", "BTimer"})  [unwired: 2 in, 2 out]
          n167 = property on="STI" class="Enum (strict)"() -> ("Value"=w166:T2)  [unwired: 2 in, 2 out]
          n168 = case shown="\"BTimer\"" w165 {
            frame "BTimer" {
              n169 = property on="btime[ms]" class="DigNum (strict)"("DisabledEnum"=i8 0) -> ()  [unwired: 2 in, 2 out]
            }
            frame Default {
              n170 = property on="btime[ms]" class="DigNum (strict)"("DisabledEnum"=i8 2) -> ()  [unwired: 2 in, 2 out]
            }
          }
          n171 = case shown="Default" w166 {
            frame "STimer" {
              n172 = property on="stime[ms]" class="DigNum (strict)"("DisabledEnum"=i8 0) -> ()  [unwired: 2 in, 2 out]
            }
            frame Default {
              n173 = property on="stime[ms]" class="DigNum (strict)"("DisabledEnum"=i8 2) -> ()  [unwired: 2 in, 2 out]
            }
          }
          n174 = global read "Globals.vi" "FFT"() -> (w164:bool)
          n175 = case shown="True" w164 {
            tunnel: [u8 0 w186] -> w167
            frame False {
            }
            frame True {
              n176 = property on="FFT mode" class="Enum (strict)"() -> ("Value"=w187:T1)  [unwired: 2 in, 2 out]
              n177 = case shown="\"Full Binning\", Default" w187 {
                tunnel: [i8 0 i8 2] -> w186
                frame "Full Binning", Default {
                }
                frame "Region of Interest", "Area" {
                }
              }
            }
          }
          n178 = property on="no.of samples (nos)" class="DigNum (strict)"("DisabledEnum"=w167) -> ()  [unwired: 2 in, 2 out]
          n179 = global read "Globals.vi" "camera system select"() -> (w162:u32)
          n180 = property on="Board select" class="CmbBox"("DisabledEnum"=w163) -> ()  [unwired: 2 in, 2 out]
          n181 = property on="Initialize" class="Bool (strict)"("DisabledEnum"=w163) -> ()  [unwired: 2 in, 2 out]
          n182 = property on="Gain" class="Bool (strict)"("DisabledEnum"=w163) -> ()  [unwired: 2 in, 2 out]
          n183 = property on="BTSlope" class="Enum (strict)"("DisabledEnum"=w163) -> ()  [unwired: 2 in, 2 out]
          n184 = property on="STSlope" class="Enum (strict)"("DisabledEnum"=w163) -> ()  [unwired: 2 in, 2 out]
          n185 = property on="is FFT" class="Bool (strict)"("DisabledEnum"=w163) -> ()  [unwired: 2 in, 2 out]
          n186 = case shown="2" w162 {
            frame 0, Default {
              n187 = property on="value white" class="DigNum (strict)"("Value"=u32 65535) -> ()  [unwired: 2 in, 2 out]
              n188 = property on="value black" class="DigNum (strict)"("Value"=u32 0) -> ()  [unwired: 2 in, 2 out]
            }
            frame 1 {
              n189 = property on="value black" class="DigNum (strict)"("Value"=u32 0) -> ()  [unwired: 2 in, 2 out]
              n190 = property on="value white" class="DigNum (strict)"("Value"=u32 65535) -> ()  [unwired: 2 in, 2 out]
            }
            frame 2 {
              n191 = property on="value black" class="DigNum (strict)"("Value"=u32 0) -> ()  [unwired: 2 in, 2 out]
              n192 = property on="value white" class="DigNum (strict)"("Value"=u32 16383) -> ()  [unwired: 2 in, 2 out]
            }
          }
          n193 = property on="fast test\ncontinuous" class="Bool (strict)"("Value"=FALSE) -> ()  [unwired: 2 in, 2 out]
          n194 = property on="BTI" class="Enum (strict)"("DisabledEnum"=w163) -> ()  [unwired: 2 in, 2 out]
          n195 = property on="STI" class="Enum (strict)"("DisabledEnum"=w163) -> ()  [unwired: 2 in, 2 out]
          n196 = property on="CC trigger" class="Enum (strict)"("DisabledEnum"=w163) -> ()  [unwired: 2 in, 2 out]
          n197 = property on="FFT mode" class="Enum (strict)"("DisabledEnum"=w163) -> ()  [unwired: 2 in, 2 out]
        }
        frame #5 {
          # "set global vars"
          n198 = global read "Globals.vi" "boards"() -> (w213:u32)
          n199 = property on="no.of blocks (nob)" class="DigNum (strict)"() -> ("Value"=w211:u32)  [unwired: 2 in, 2 out]
          n200 = property on="no.of samples (nos)" class="DigNum (strict)"() -> ("Value"=w212:u32)  [unwired: 2 in, 2 out]
          n201 = case shown="2" w213 {
            frame 1, Default {
              n202 = global write "Globals.vi" "board_sel"(u32 1) -> ()
            }
            frame 2 {
              n203 = case shown="\"both boards\"" "Board select" {
                frame "board 2" {
                  n204 = global write "Globals.vi" "board_sel"(u32 2) -> ()
                }
                frame "both boards" {
                  n205 = global write "Globals.vi" "board_sel"(u32 3) -> ()
                }
                frame "board 1", Default {
                  n206 = global write "Globals.vi" "board_sel"(u32 1) -> ()
                }
              }
            }
          }
          n207 = global write "Globals.vi" "nos"(w212) -> ()
          n208 = global write "Globals.vi" "nob"(w211) -> ()
          n209 = global write "Globals.vi" "STSlope"("STSlope") -> ()
          n210 = global write "Globals.vi" "BTSlope"("BTSlope") -> ()
          n211 = global write "Globals.vi" "CCtrigger"("CC trigger") -> ()
          n212 = global write "Globals.vi" "Gain"("Gain") -> ()
          n213 = property on="SDAT in 10ns" class="DigNum (strict)"() -> ("Value"=w208:u32)  [unwired: 2 in, 2 out]
          n214 = global write "Globals.vi" "BTI"("BTI") -> ()
          n215 = global write "Globals.vi" "STI"("STI") -> ()
          n216 = property on="btime[ms]" class="DigNum (strict)"() -> ("Value"=w209:dbl)  [unwired: 2 in, 2 out]
          n217 = property on="stime[ms]" class="DigNum (strict)"() -> ("Value"=w210:dbl)  [unwired: 2 in, 2 out]
          n218 = property on="DAC 3/ 1" class="DigNum (strict)"() -> ("Value"=w205:u16)  [unwired: 2 in, 2 out]
          n219 = property on="DAC 4/ 1" class="DigNum (strict)"() -> ("Value"=w204:u16)  [unwired: 2 in, 2 out]
          n220 = property on="DAC 5/ 1" class="DigNum (strict)"() -> ("Value"=w203:u16)  [unwired: 2 in, 2 out]
          n221 = property on="DAC 2/ 1" class="DigNum (strict)"() -> ("Value"=w206:u16)  [unwired: 2 in, 2 out]
          n222 = property on="DAC 1/ 1" class="DigNum (strict)"() -> ("Value"=w207:u16)  [unwired: 2 in, 2 out]
          n223 = global write "Globals.vi" "SDAT in 100ns"(w208) -> ()
          n224 = global write "Globals.vi" "btime[ms]"(w209) -> ()
          n225 = global write "Globals.vi" "stime[ms]"(w210) -> ()
          n226 = global write "Globals.vi" "DAC1"(w206) -> ()
          n227 = global write "Globals.vi" "DAC4"(w203) -> ()
          n228 = global write "Globals.vi" "DAC0"(w207) -> ()
          n229 = global write "Globals.vi" "DAC2"(w205) -> ()
          n230 = global write "Globals.vi" "DAC3"(w204) -> ()
          n231 = property on="DAC 6/ 1" class="DigNum (strict)"() -> ("Value"=w202:u16)  [unwired: 2 in, 2 out]
          n232 = property on="DAC 8/ 1" class="DigNum (strict)"() -> ("Value"=w201:u16)  [unwired: 2 in, 2 out]
          n233 = property on="DAC 7/ 1" class="DigNum (strict)"() -> ("Value"=w200:u16)  [unwired: 2 in, 2 out]
          n234 = property on="cool" class="DigNum (strict)"() -> ("Value"=w198:u8)  [unwired: 2 in, 2 out]
          n235 = global write "Globals.vi" "DAC5"(w202) -> ()
          n236 = global write "Globals.vi" "DAC6"(w200) -> ()
          n237 = global write "Globals.vi" "DAC7"(w201) -> ()
          n238 = global write "Globals.vi" "cool level"(w198) -> ()
        }
        frame #6 {
          n239 = call "InitBrd_multicam.vi"() -> ("error out"=w225:errorcluster)  [unwired: 10 in]
          n240 = call "InitMeasurement.vi"("error in (no error)"=w225) -> ("error out"=w224:errorcluster)  [unwired: 10 in]
          n241 = call <vilib>:"Simple Error Handler.vi"("error in (no error)"=w224) -> ()  [unwired: 4 in, 5 out]
        }
      }
    }
    frame #2 {
      w229 = FALSE
      w231 = 2
      # "cosmetics of the graphs for more cams"
      n242 = property on="framewise\ncontinuous" class="Bool (strict)"("DisabledEnum"=w231) -> ()  [unwired: 2 in, 2 out]
      n243 = property on="block" class="Slide (strict)"("DisabledEnum"=w231) -> ()  [unwired: 2 in, 2 out]
      n244 = property on="fast test\ncontinuous" class="Bool (strict)"("DisabledEnum"=w231) -> ()  [unwired: 2 in, 2 out]
      n245 = property on="start" class="Bool (strict)"("DisabledEnum"=w231) -> ()  [unwired: 2 in, 2 out]
      n246 = property on="sample" class="Slide (strict)"("DisabledEnum"=w231) -> ()  [unwired: 2 in, 2 out]
      n247 = property on="exit" class="Bool (strict)"("DisabledEnum"=0) -> ()  [unwired: 2 in, 2 out]
      n248 = Boolean To (0,1)(Boolean=w229) -> (0, 1=w228:i16)
      n249 = property on="Measure on" class="Bool (strict)"("Value"=w229) -> ()  [unwired: 2 in, 2 out]
      n250 = To Unsigned Byte Integer(number=w228) -> (unsigned 8bit integer=w227:u8)
      n251 = property on="framewise\ncontinuous" class="Bool (strict)"("Value"=w229) -> ()  [unwired: 2 in, 2 out]
      n252 = call "contFFLoop.vi"("pause"=u32 1, "activate"=w227) -> ()  [unwired: 8 in, 1 out]
      n253 = global read "Globals.vi" "boards"() -> (w230:u32)
      n254 = case shown="2" w230 {
        frame 2 {
          n255 = global read "Globals.vi" "CAMCNT"() -> (w237:u32)
          n256 = case shown="1, Default" w237 {
            tunnel: [TRUE w244 w245 w247] -> w236
            tunnel: [w241 w244 w245 w247] -> w235
            tunnel: [w241 FALSE w245 w247] -> w234
            frame 2 {
              w241 = FALSE
              n257 = property on="Signal Board 1 / Cam 1" class="WFGraph (strict)"("Height"=u32 170) -> ()  [unwired: 2 in, 2 out]
            }
            frame 3 {
              w244 = TRUE
            }
            frame 4 {
              w245 = TRUE
            }
            frame 1, Default {
              w247 = FALSE
              n258 = property on="Signal Board 1 / Cam 1" class="WFGraph (strict)"("Height"=u32 170) -> ()  [unwired: 2 in, 2 out]
              n259 = property on="Signal Board 1 / Cam1" class="WFGraph (strict)"("Top"=0) -> ()  [unwired: 2 in, 2 out]
            }
          }
          n260 = property on="Signal Board 1 / Cam1" class="WFGraph (strict)"("Height"=u32 170) -> ()  [unwired: 2 in, 2 out]
          n261 = property on="Signal Board 2 / Cam1" class="WFGraph (strict)"("Visible"=TRUE) -> ()  [unwired: 2 in, 2 out]
          n262 = property on="Signal Board 1 / Cam 3" class="WFGraph (strict)"("Visible"=w235) -> ()  [unwired: 2 in, 2 out]
          n263 = property on="Signal Board 1 / Cam 4" class="WFGraph (strict)"("Visible"=w234) -> ()  [unwired: 2 in, 2 out]
          n264 = property on="Signal Board 1 / Cam 2" class="WFGraph (strict)"("Visible"=w236) -> ()  [unwired: 2 in, 2 out]
        }
        frame 1, Default {
          n265 = global read "Globals.vi" "CAMCNT"() -> (w252:u32)
          n266 = case shown="2" w252 {
            tunnel: [TRUE w262 w267 w268] -> w251
            tunnel: [w256 w262 w267 w268] -> w250
            tunnel: [w256 FALSE w267 w268] -> w249
            frame 2 {
              w256 = FALSE
              n267 = property on="Signal Board 1 / Cam1" class="WFGraph (strict)"("Height"=u32 170) -> ()  [unwired: 2 in, 2 out]
              n268 = property on="Signal Cam 2" class="WFGraph (strict)"("Top"=250) -> ()  [unwired: 2 in, 2 out]
            }
            frame 3 {
              w262 = TRUE
              n269 = property on="Signal Board 1 / Cam1" class="WFGraph (strict)"("Height"=u32 170) -> ()  [unwired: 2 in, 2 out]
              n270 = property on="Signal Cam 2" class="WFGraph (strict)"("Top"=250) -> ()  [unwired: 2 in, 2 out]
              n271 = property on="Signal Cam 3" class="WFGraph (strict)"("Top"=-250) -> ()  [unwired: 2 in, 2 out]
            }
            frame 4 {
              w267 = TRUE
              n272 = property on="Signal Board 1 / Cam1" class="WFGraph (strict)"("Height"=u32 170) -> ()  [unwired: 2 in, 2 out]
              n273 = property on="Signal Cam 3" class="WFGraph (strict)"("Top"=-250) -> ()  [unwired: 2 in, 2 out]
              n274 = property on="Signal Cam 2" class="WFGraph (strict)"("Top"=250) -> ()  [unwired: 2 in, 2 out]
              n275 = property on="Signal Cam 4" class="WFGraph (strict)"("Top"=-500) -> ()  [unwired: 2 in, 2 out]
            }
            frame 1, Default {
              w268 = FALSE
              n276 = property on="Signal Board 1 / Cam1" class="WFGraph (strict)"("Height"=u32 400) -> ()  [unwired: 2 in, 2 out]
            }
          }
          n277 = property on="Signal Board 2 / Cam1" class="WFGraph (strict)"("Visible"=FALSE) -> ()  [unwired: 2 in, 2 out]
          n278 = property on="Signal Cam 3" class="WFGraph (strict)"("Visible"=w250) -> ()  [unwired: 2 in, 2 out]
          n279 = property on="Signal Cam 4" class="WFGraph (strict)"("Visible"=w249) -> ()  [unwired: 2 in, 2 out]
          n280 = property on="Signal Cam 2" class="WFGraph (strict)"("Visible"=w251) -> ()  [unwired: 2 in, 2 out]
        }
      }
      n281 = property on="# boards \ndetected" class="DigNum (strict)"("Visible"=TRUE) -> ()  [unwired: 2 in, 2 out]
    }
    frame #3 {
      # "display / hide chosen labview elements"
      n282 = global read "Globals.vi" "debug_mode"() -> (w276:bool)
      n283 = global read "Globals.vi" "camera system select"() -> (w273:u32)
      n284 = case shown="2" w273 {
        tunnel: [FALSE FALSE TRUE] -> w274
        frame 0, Default {
        }
        frame 1 {
        }
        frame 2 {
        }
      }
      n285 = And(x=w274, y=w276) -> (x .and. y?=w271:bool)
      n286 = property on="custom patt: 14bits pattern hex (14bit)" class="DigNum (strict)"("Visible"=w271) -> ()  [unwired: 2 in, 2 out]
      n287 = property on="ADC mode" class="RadioBtnsControl (strict)"("Visible"=w271) -> ()  [unwired: 2 in, 2 out]
      n288 = property on="pattern dec" class="DigNum (strict)"("Visible"=w271) -> ()  [unwired: 2 in, 2 out]
      n289 = global read "Globals.vi" "use DAC"() -> (w275:bool)
      n290 = And(x=w274, y=w275) -> (x .and. y?=w270:bool)
      n291 = property on="DAC 3/ 1" class="DigNum (strict)"("Visible"=w270) -> ()  [unwired: 2 in, 2 out]
      n292 = property on="DAC 5/ 1" class="DigNum (strict)"("Visible"=w270) -> ()  [unwired: 2 in, 2 out]
      n293 = property on="DAC 4/ 1" class="DigNum (strict)"("Visible"=w270) -> ()  [unwired: 2 in, 2 out]
      n294 = property on="DAC 6/ 1" class="DigNum (strict)"("Visible"=w270) -> ()  [unwired: 2 in, 2 out]
      n295 = property on="DAC 7/ 1" class="DigNum (strict)"("Visible"=w270) -> ()  [unwired: 2 in, 2 out]
      n296 = property on="DAC 8/ 1" class="DigNum (strict)"("Visible"=w270) -> ()  [unwired: 2 in, 2 out]
      n297 = property on="DAC 1/ 1" class="DigNum (strict)"("Visible"=w270) -> ()  [unwired: 2 in, 2 out]
      n298 = property on="Offset" class="Bool (strict)"("Visible"=w270) -> ()  [unwired: 2 in, 2 out]
      n299 = property on="DAC 2/ 1" class="DigNum (strict)"("Visible"=w270) -> ()  [unwired: 2 in, 2 out]
      n300 = property on="Offset" class="Bool (strict)"() -> ("Value"=w272:bool)  [unwired: 2 in, 2 out]
      n301 = property on="Offset" class="Bool (strict)"("Val(Sgnl)"=w272) -> ()  [unwired: 2 in, 2 out]
    }
    frame #4 {
      # "event structure while running"
      n302 = while {
        tunnel: w280 -> [w281]
        stop <- w283 stop-if-true
        w282 = 25
        # "event \ntimeout"
        n303 = event shown="[6] \"startevent\": Value Change" {
          selector: w281 -> [_ _ _ _ _ _ _ _ _ _ _ _ _ _ _ _ _ _ _ _ _ _ _ _ _ _ _ _ _]
          dyn-events: _ -> [_ _ _ _ _ _ _ _ _ _ _ _ _ _ _ _ _ _ _ _ _ _ _ _ _ _ _ _ _]
          timeout: w282 -> [_ _ _ _ _ _ _ _ _ _ _ _ _ _ _ _ _ _ _ _ _ _ _ _ _ _ _ _ _]
          tunnel: [_ _ _ _ _ _ _ _ _ _ _ _ _ _ _ _ w512 _ _ _ _ _ _ _ _ _ _ _ _] -> w283
          tunnel: w282 -> [_ w327 _ _ _ _ _ _ _ _ _ _ _ _ _ _ _ _ _ _ _ _ _ _ _ _ _ _ _]
          event Timeout; "refresh": Value Change {
            w291 = u32 0
            w312 = u32 1
            # "only refresh the frames if measure on"
            # "timout excecutes every 100ms"
            # "userinfo of RAM, MeasureOB and setting display event in cont mode"
            n304 = event-data() -> ()  [unwired: 1 in, 3 out]
            n305 = call "FreeMemInfo.vi"() -> ("PhysicalFreeSpace"=→"FREE \nRAM MB":dbl, "PhysicalSpace"=→"BUILT-IN\nRAM MB":dbl)  [unwired: 8 in, 1 out]
            n306 = property on="Measure on" class="Bool (strict)"() -> ("Value"=w286:bool)  [unwired: 2 in, 2 out]
            n307 = property on="framewise\ncontinuous" class="Bool (strict)"() -> ("DisabledEnum"=w316:T4)  [unwired: 2 in, 2 out]
            n308 = property on="no.of samples (nos)" class="DigNum (strict)"() -> ("Value"=w285:u32)  [unwired: 2 in, 2 out]
            n309 = case shown="False" w286 {
              tunnel: [2 0] -> w288
              frame False {
              }
              frame True {
              }
            }
            n310 = property on="no.of blocks (nob)" class="DigNum (strict)"() -> ("Value"=w284:u32)  [unwired: 2 in, 2 out]
            n311 = property on="(LastCAM) \n        C1" class="Bool (strict)"("DisabledEnum"=w288) -> ()  [unwired: 2 in, 2 out]
            n312 = property on="C 2" class="Bool (strict)"("DisabledEnum"=w288) -> ()  [unwired: 2 in, 2 out]
            n313 = property on="C 3" class="Bool (strict)"("DisabledEnum"=w288) -> ()  [unwired: 2 in, 2 out]
            n314 = property on="C 4" class="Bool (strict)"("DisabledEnum"=w288) -> ()  [unwired: 2 in, 2 out]
            n315 = property on="framewise\ncontinuous" class="Bool (strict)"() -> ("Value"=w290:bool)  [unwired: 2 in, 2 out]
            n316 = Equal?(x=w284, y=w312) -> (x = y?=w310:bool)
            n317 = Equal?(x=w312, y=w285) -> (x = y?=w311:bool)
            n318 = property on="C 5" class="Bool (strict)"("DisabledEnum"=w288) -> ()  [unwired: 2 in, 2 out]
            n319 = property on="C 6" class="Bool (strict)"("DisabledEnum"=w288) -> ()  [unwired: 2 in, 2 out]
            n320 = property on="C 7" class="Bool (strict)"("DisabledEnum"=w288) -> ()  [unwired: 2 in, 2 out]
            n321 = property on="C 8" class="Bool (strict)"("DisabledEnum"=w288) -> ()  [unwired: 2 in, 2 out]
            n322 = To Unsigned Byte Integer(number=w316) -> (unsigned 8bit integer=w317:u8)
            n323 = And(x=w310, y=w311) -> (x .and. y?=w309:bool)
            n324 = Equal?(x=w317, y=u8 0) -> (x = y?=w289:bool)
            n325 = property on="Measure on" class="Bool (strict)"() -> ("Value"=w287:bool)  [unwired: 2 in, 2 out]
            n326 = And(x=w290, y=w289) -> (x .and. y?=w314:bool)
            n327 = Or(x=w309, y=w314) -> (x .or. y?=w313:bool)
            n328 = call "BitTest.vi"("BitAddr"=u32 8, "Offset"=w291) -> ("Bool Board 1"=→"(LastCAM) \n        C1":bool)  [unwired: 6 in, 2 out]
            n329 = call "BitTest.vi"("BitAddr"=u32 9, "Offset"=w291) -> ("Bool Board 1"=→"C 2":bool)  [unwired: 6 in, 2 out]
            n330 = call "BitTest.vi"("BitAddr"=u32 10, "Offset"=w291) -> ("Bool Board 1"=→"C 3":bool)  [unwired: 6 in, 2 out]
            n331 = call "BitTest.vi"("BitAddr"=u32 11, "Offset"=w291) -> ("Bool Board 1"=→"C 4":bool)  [unwired: 6 in, 2 out]
            n332 = And(x=w313, y=w287) -> (x .and. y?=w315:bool)
            n333 = case shown="True" w315 {
              frame False {
              }
              frame True {
                # "trigger the \ndisplay event"
                n334 = property on="sample" class="Slide (strict)"() -> ("Value"=w323:u32)  [unwired: 2 in, 2 out]
                n335 = property on="sample" class="Slide (strict)"("Val(Sgnl)"=w323) -> ()  [unwired: 2 in, 2 out]
              }
            }
            n336 = call "ReadL.vi"("Offset"=w291) -> ("Data 1"=→"cool_temp Reg":u32)  [unwired: 8 in, 2 out]
            n337 = call "BitTest.vi"("BitAddr"=u32 12, "Offset"=w291) -> ("Bool Board 1"=→"C 5":bool)  [unwired: 6 in, 2 out]
            n338 = call "BitTest.vi"("BitAddr"=u32 13, "Offset"=w291) -> ("Bool Board 1"=→"C 6":bool)  [unwired: 6 in, 2 out]
            n339 = call "BitTest.vi"("BitAddr"=u32 14, "Offset"=w291) -> ("Bool Board 1"=→"C 7":bool)  [unwired: 6 in, 2 out]
            n340 = call "BitTest.vi"("BitAddr"=u32 15, "Offset"=w291) -> ("Bool Board 1"=→"C 8":bool)  [unwired: 6 in, 2 out]
          }
          event "framewise\ncontinuous": Value Change {
            # "Warning Message for correcting wrong exp time"
            n341 = event-data() -> ()  [unwired: 1 in, 6 out]
            n342 = Add(x=u32 20, y=w327) -> (x+y=w328:u32)
            n343 = global read "Globals.vi" "mshut"() -> (w335:bool)
            n344 = property on="BTI" class="Enum (strict)"() -> ("Value"=w331:enum32{"I", "S1", "S2", "S1&S2", "BTimer"})  [unwired: 2 in, 2 out]
            n345 = case shown="True" "framewise\ncontinuous" {
              tunnel: [u8 0 u8 1] -> w340
              tunnel: [u8 2 u8 0] -> w339
              tunnel: [FALSE FALSE] -> w337
              tunnel: [u8 0 w356] -> w338
              tunnel: [u32 1 w355] -> w329
              tunnel: w328 -> [_ w355]
              frame False {
              }
              frame True {
                n346 = property on="sample" class="Slide (strict)"() -> ("DisabledEnum"=w356:T4)  [unwired: 2 in, 2 out]
              }
            }
            n347 = property on="no.of blocks (nob)" class="DigNum (strict)"("DisabledEnum"=w338) -> ()  [unwired: 2 in, 2 out]
            n348 = property on="sample" class="Slide (strict)"("DisabledEnum"=w338) -> ()  [unwired: 2 in, 2 out]
            n349 = property on="block" class="Slide (strict)"("DisabledEnum"=w338) -> ()  [unwired: 2 in, 2 out]
            n350 = global read "Globals.vi" "FFT"() -> (w324:bool)
            n351 = case shown="\"BTimer\"" w331 {
              tunnel: [TRUE FALSE] -> w330
              frame "BTimer" {
              }
              frame Default {
              }
            }
            n352 = Not(x=w335) -> (.not. x?=w334:bool)
            n353 = property on="alloc mem" class="Bool (strict)"("DisabledEnum"=w338) -> ()  [unwired: 2 in, 2 out]
            n354 = And(x=w324, y=w334) -> (x .and. y?=w333:bool)
            n355 = call "contFFLoop.vi"("pause"=w329, "activate"=w340) -> ()  [unwired: 8 in, 1 out]
            n356 = And(x=w333, y=w330) -> (x .and. y?=w332:bool)
            n357 = case shown="True" w332 {
              tunnel: [FALSE w345] -> w336
              frame False {
              }
              frame True {
                n358 = property on="FFT mode" class="Enum (strict)"() -> ("Value"=w346:T1)  [unwired: 2 in, 2 out]
                n359 = case shown="Default" w346 {
                  tunnel: [FALSE w348] -> w345
                  frame Default {
                  }
                  frame "Region of Interest", "Area" {
                    n360 = property on="framewise\ncontinuous" class="Bool (strict)"() -> ("Value"=w348:bool)  [unwired: 2 in, 2 out]
                  }
                }
              }
            }
            n361 = property on="fast test\ncontinuous" class="Bool (strict)"("DisabledEnum"=w339) -> ()  [unwired: 2 in, 2 out]
            n362 = property on="fast test\ncontinuous" class="Bool (strict)"("Value"=w337) -> ()  [unwired: 2 in, 2 out]
            n363 = global read "Globals.vi" "FFT"() -> (w325:bool)
            n364 = case shown="False" w325 {
              tunnel: w338 -> [w349 _]
              frame False {
                n365 = property on="no.of samples (nos)" class="DigNum (strict)"("DisabledEnum"=w349) -> ()  [unwired: 2 in, 2 out]
              }
              frame True {
              }
            }
            n366 = property on="String" class="Str"("Blinking"=w336) -> ()  [unwired: 2 in, 2 out]
            n367 = property on="String" class="Str"("Visible"=w336) -> ()  [unwired: 2 in, 2 out]
          }
          event "fast test\ncontinuous": Value Change {
            # "2 because with 1 the old \ncont mode is set"
            # "setting fast continuos mode"
            n368 = event-data() -> ()  [unwired: 1 in, 6 out]
            n369 = case shown="True" "fast test\ncontinuous" {
              tunnel: [0 2] -> w361
              frame False {
                n370 = property on="no.of samples (nos)" class="DigNum (strict)"() -> ("Value"=w364:u32)  [unwired: 2 in, 2 out]
                n371 = property on="alloc mem" class="Bool (strict)"() -> ("Value"=w365:bool)  [unwired: 2 in, 2 out]
                n372 = property on="alloc mem" class="Bool (strict)"("Val(Sgnl)"=w365) -> ()  [unwired: 2 in, 2 out]
                n373 = property on="no.of samples (nos)" class="DigNum (strict)"("Val(Sgnl)"=w364) -> ()  [unwired: 2 in, 2 out]
              }
              frame True {
                n374 = property on="FFT mode" class="Enum (strict)"() -> ("Value"=w367:T1)  [unwired: 2 in, 2 out]
                n375 = property on="stime[ms]" class="DigNum (strict)"() -> ("Value"=w368:dbl)  [unwired: 2 in, 2 out]
                n376 = case shown="Default" w367 {
                  tunnel: w368 -> [_ w372]
                  frame "Region of Interest", "Area" {
                    n377 = property on="no.of samples (nos)" class="DigNum (strict)"() -> ("Value"=w370:u32)  [unwired: 2 in, 2 out]
                    n378 = global write "Globals.vi" "nos"(w370) -> ()
                  }
                  frame Default {
                    w377 = u32 2
                    n379 = Divide(x=u32 50, y=w372) -> (x/y=w374:dbl)
                    n380 = To Unsigned Long Integer(number=w374) -> (unsigned 32bit integer=w376:u32)
                    n381 = Less?(x=w376, y=w377) -> (x < y?=w375:bool)
                    n382 = case shown="False" w375 {
                      tunnel: w376 -> [w378 _]
                      tunnel: [w378 w379] -> w371
                      tunnel: w377 -> [_ w379]
                      frame False {
                      }
                      frame True {
                      }
                    }
                    n383 = property on="sample" class="Slide (strict)"("Value"=w371) -> ()  [unwired: 2 in, 2 out]
                    n384 = property on="no.of samples (nos)" class="DigNum (strict)"("Value"=w371) -> ()  [unwired: 2 in, 2 out]
                    n385 = global write "Globals.vi" "nos"(w371) -> ()
                  }
                }
                n386 = call "SetMeasurementParameters.vi"() -> ()  [unwired: 11 in, 1 out]
              }
            }
            n387 = property on="no.of blocks (nob)" class="DigNum (strict)"("DisabledEnum"=w361) -> ()  [unwired: 2 in, 2 out]
            n388 = property on="alloc mem" class="Bool (strict)"("DisabledEnum"=w361) -> ()  [unwired: 2 in, 2 out]
            n389 = property on="sample" class="Slide (strict)"("DisabledEnum"=w361) -> ()  [unwired: 2 in, 2 out]
            n390 = global read "Globals.vi" "FFT"() -> (w360:bool)
            n391 = property on="block" class="Slide (strict)"("DisabledEnum"=w361) -> ()  [unwired: 2 in, 2 out]
            n392 = case shown="False" w360 {
              tunnel: w361 -> [w363 _]
              frame False {
                n393 = property on="no.of samples (nos)" class="DigNum (strict)"("DisabledEnum"=w363) -> ()  [unwired: 2 in, 2 out]
              }
              frame True {
              }
            }
          }
          event "alloc mem": Mouse Down {
            w383 = 0
            # "trigger dac update"
            # "update params"
            n394 = event-data() -> ()  [unwired: 1 in, 8 out]
            n395 = property on="no.of samples (nos)" class="DigNum (strict)"() -> ("Value"=w381:u32)  [unwired: 2 in, 2 out]
            n396 = property on="no.of blocks (nob)" class="DigNum (strict)"() -> ("Value"=w380:u32)  [unwired: 2 in, 2 out]
            n397 = property on="send all" class="Bool (strict)"() -> ("Value"=w384:bool)  [unwired: 2 in, 2 out]
            n398 = global write "Globals.vi" "nob"(w380) -> ()
            n399 = global write "Globals.vi" "nos"(w381) -> ()
            n400 = property on="send all" class="Bool (strict)"("Val(Sgnl)"=w384) -> ()  [unwired: 2 in, 2 out]
            n401 = call "SetMeasurementParameters.vi"() -> ()  [unwired: 11 in, 1 out]
            n402 = property on="show greyscale viewer" class="Bool (strict)"("DisabledEnum"=0) -> ()  [unwired: 2 in, 2 out]
            n403 = property on="stime[ms]" class="DigNum (strict)"() -> ("Value"=w386:dbl)  [unwired: 2 in, 2 out]
            n404 = property on="TRMS Pix" class="DigNum (strict)"("DisabledEnum"=w383) -> ()  [unwired: 2 in, 2 out]
            n405 = property on="SDAT in 10ns" class="DigNum (strict)"() -> ("Value"=w385:u32)  [unwired: 2 in, 2 out]
            n406 = property on="start" class="Bool (strict)"("DisabledEnum"=w383) -> ()  [unwired: 2 in, 2 out]
            n407 = property on="sample" class="Slide (strict)"("DisabledEnum"=w383) -> ()  [unwired: 2 in, 2 out]
            n408 = property on="framewise\ncontinuous" class="Bool (strict)"("DisabledEnum"=w383) -> ()  [unwired: 2 in, 2 out]
            n409 = property on="block" class="Slide (strict)"("DisabledEnum"=w383) -> ()  [unwired: 2 in, 2 out]
            n410 = property on="stime[ms]" class="DigNum (strict)"("Val(Sgnl)"=w386) -> ()  [unwired: 2 in, 2 out]
            n411 = property on="SDAT in 10ns" class="DigNum (strict)"("Val(Sgnl)"=w385) -> ()  [unwired: 2 in, 2 out]
          }
          event "show greyscale viewer": Value Change {
            n412 = event-data() -> ()  [unwired: 1 in, 6 out]
            n413 = case shown="True" "show greyscale viewer" {
              frame False {
                n414 = call "deinit2dViewer.vi"() -> ()  [unwired: 11 in, 1 out]
              }
              frame True {
                n415 = flat-sequence {
                  frame #0 {
                    n416 = property on="no.of samples (nos)" class="DigNum (strict)"() -> ("Value"=w388:u32)  [unwired: 2 in, 2 out]
                    n417 = call "show2dViewer.vi"("nos"=w388, "cam"=u16 0, "cur_nob"=u16 0) -> ()  [unwired: 8 in, 1 out]
                  }
                  frame #1 {
                    n418 = property on="value black" class="DigNum (strict)"() -> ("Value"=w393:u32)  [unwired: 2 in, 2 out]
                    n419 = property on="sample" class="Slide (strict)"() -> ("Value"=w391:u32)  [unwired: 2 in, 2 out]
                    n420 = property on="value white" class="DigNum (strict)"() -> ("Value"=w392:u32)  [unwired: 2 in, 2 out]
                    n421 = call "setGamma.vi"("black"=w393, "white"=w392) -> ()  [unwired: 10 in]
                    n422 = property on="sample" class="Slide (strict)"("Val(Sgnl)"=w391) -> ()  [unwired: 2 in, 2 out]
                  }
                }
              }
            }
          }
          event "start": Mouse Down {
            # "start measurement"
            n423 = event-data() -> ()  [unwired: 1 in, 8 out]
            n424 = property on="startevent" class="Bool (strict)"("Val(Sgnl)"="startevent") -> ()  [unwired: 2 in, 2 out]
            n425 = property on="refresh" class="Bool (strict)"("Val(Sgnl)"="refresh") -> ()  [unwired: 2 in, 2 out]
            n426 = case shown="True" FALSE {
              frame False {
              }
              frame True {
                w398 = u8 5 items=["S0Addr_CtrlA"=4, "S0Addr_CtrlB"=5, "S0Addr_CtrlC"=6, "S0Addr_XCKLL"=8, "S0Addr_XCKLH"=9, "S0Addr_XCKHL"=10, "S0Addr_XCKMSB"=11, "S0Addr_XCKCNTLL"=12, "S0Addr_XCKCNTLH"=13, "S0Addr_XCKCNTHL"=14, "S0Addr_XCKCNTMSB"=15, "S0Addr_PIXREGlow"=16, "S0Addr_PIXREGhigh"=17, "S0Addr_FREQREG"=18, "S0Addr_FF_FLAGS"=19, "S0Addr_FIFOCNT"=20, "S0Addr_VCLKCTRL"=24, "S0Addr_EBST"=28, "S0Addr_DAT"=32, "S0Addr_EC"=36, "S0Addr_TOR"=40, "S0Addr_ARREG"=44, "S0Addr_GIOREG"=48, "S0Addr_DELAYEC"=52, "S0Addr_IRQREG"=56, "S0Addr_PCI"=60]
                # "CtrlB register @ 0x05"
                n427 = call "WriteB.vi"("val"=u8 33, "offset"=w398) -> ()  [unwired: 9 in, 1 out]
              }
            }
            n428 = property on="Offset" class="Bool (strict)"() -> ("Value"=w397:bool)  [unwired: 2 in, 2 out]
            n429 = case shown="True" w397 {
              frame False {
                n430 = global write "Globals.vi" "board_sel_offset"(u32 1) -> ()
              }
              frame True {
                n431 = global write "Globals.vi" "board_sel_offset"(u32 2) -> ()
              }
            }
          }
          event "startevent": Value Change {
            n432 = event-data() -> ()  [unwired: 1 in, 6 out]
            n433 = call "ReadFFLoop_thread.vi"() -> ()  [unwired: 11 in, 1 out]
          }
          event "start": Mouse Up {
            w402 = 0
            # "refresh trms and signalgraph if measurtime is too short for the Measure On LED (<100ms / Timeout)"
            n434 = event-data() -> ()  [unwired: 1 in, 8 out]
            n435 = property on="DAC 3/ 1" class="DigNum (strict)"("DisabledEnum"=w402) -> ()  [unwired: 2 in, 2 out]
            n436 = property on="DAC 1/ 1" class="DigNum (strict)"("DisabledEnum"=w402) -> ()  [unwired: 2 in, 2 out]
            n437 = property on="DAC 2/ 1" class="DigNum (strict)"("DisabledEnum"=w402) -> ()  [unwired: 2 in, 2 out]
            n438 = property on="DAC 4/ 1" class="DigNum (strict)"("DisabledEnum"=w402) -> ()  [unwired: 2 in, 2 out]
            n439 = property on="TRMS Pix" class="DigNum (strict)"() -> ("Value"=w405:u32)  [unwired: 2 in, 2 out]
            n440 = property on="Pixel for Graph" class="Slide (strict)"() -> ("Value"=w403:u32)  [unwired: 2 in, 2 out]
            n441 = property on="sample" class="Slide (strict)"() -> ("Value"=w404:u32)  [unwired: 2 in, 2 out]
            n442 = property on="DAC 6/ 1" class="DigNum (strict)"("DisabledEnum"=w402) -> ()  [unwired: 2 in, 2 out]
            n443 = property on="DAC 7/ 1" class="DigNum (strict)"("DisabledEnum"=w402) -> ()  [unwired: 2 in, 2 out]
            n444 = property on="DAC 5/ 1" class="DigNum (strict)"("DisabledEnum"=w402) -> ()  [unwired: 2 in, 2 out]
            n445 = property on="DAC 8/ 1" class="DigNum (strict)"("DisabledEnum"=w402) -> ()  [unwired: 2 in, 2 out]
            n446 = property on="TRMS Pix" class="DigNum (strict)"("Val(Sgnl)"=w405) -> ()  [unwired: 2 in, 2 out]
            n447 = property on="Pixel for Graph" class="Slide (strict)"("Val(Sgnl)"=w403) -> ()  [unwired: 2 in, 2 out]
            n448 = property on="sample" class="Slide (strict)"("Val(Sgnl)"=w404) -> ()  [unwired: 2 in, 2 out]
            n449 = property on="Offset" class="Bool (strict)"("DisabledEnum"=w402) -> ()  [unwired: 2 in, 2 out]
            n450 = property on="send all" class="Bool (strict)"("DisabledEnum"=w402) -> ()  [unwired: 2 in, 2 out]
          }
          event "sample", "block": Value Change {
            n451 = event-data() -> ()  [unwired: 1 in, 6 out]
            n452 = stacked-sequence {
              frame #0 {
                w419 = u32 1
                # "display"
                n453 = Subtract(x="sample", y=w419) -> (x-y=w414:u32)
                n454 = Subtract(x="block", y=w419) -> (x-y=w411:u32)
                n455 = global read "Globals.vi" "CAMCNT"() -> (w418:u32)
                n456 = case shown="1, Default" w418 {
                  tunnel: w411 -> [_ w431 w437 w449]
                  tunnel: w414 -> [_ w426 w436 w448]
                  tunnel: [w420 w424 w432 w442] -> w417
                  tunnel: [w420 w427 w433 w443] -> w416
                  tunnel: [w420 w427 w438 w444] -> w415
                  frame 1, Default {
                    n457 = To Long Integer(number=u16 1088) -> (32bit integer=w421:i32)
                    n458 = Initialize Array(u16 0, w421) -> (w420:u16[])
                  }
                  frame 2 {
                    n459 = To Long Integer(number=u16 1088) -> (32bit integer=w428:i32)
                    n460 = Initialize Array(u16 0, w428) -> (w427:u16[])
                    n461 = call "ReturnFrame.vi"("curr_nob"=w431, "curr_nos"=w426, "curr_cam"=u16 1) -> ("Data Values Out 1"=w424:u16[])  [unwired: 6 in, 2 out]
                  }
                  frame 3 {
                    n462 = To Long Integer(number=u16 1088) -> (32bit integer=w439:i32)
                    n463 = call "ReturnFrame.vi"("curr_nob"=w437, "curr_nos"=w436, "curr_cam"=u16 1) -> ("Data Values Out 1"=w432:u16[])  [unwired: 6 in, 2 out]
                    n464 = Initialize Array(u16 0, w439) -> (w438:u16[])
                    n465 = call "ReturnFrame.vi"("curr_nob"=w437, "curr_nos"=w436, "curr_cam"=u16 2) -> ("Data Values Out 1"=w433:u16[])  [unwired: 6 in, 2 out]
                  }
                  frame 4 {
                    n466 = call "ReturnFrame.vi"("curr_nob"=w449, "curr_nos"=w448, "curr_cam"=u16 3) -> ("Data Values Out 1"=w444:u16[])  [unwired: 6 in, 2 out]
                    n467 = call "ReturnFrame.vi"("curr_nob"=w449, "curr_nos"=w448, "curr_cam"=u16 1) -> ("Data Values Out 1"=w442:u16[])  [unwired: 6 in, 2 out]
                    n468 = call "ReturnFrame.vi"("curr_nob"=w449, "curr_nos"=w448, "curr_cam"=u16 2) -> ("Data Values Out 1"=w443:u16[])  [unwired: 6 in, 2 out]
                  }
                }
                "Signal Cam 2" <- w417
                "Signal Cam 3" <- w416
                "Signal Cam 4" <- w415
                n469 = call "ReturnFrame.vi"("curr_nob"=w411, "curr_nos"=w414, "curr_cam"=u16 0) -> ("Data Values Out 2"=→"Signal Board 2 / Cam1":u16[], "Data Values Out 1"=→"Signal Board 1 / Cam1":u16[])  [unwired: 6 in, 1 out]
                n470 = property on="no.of samples (nos)" class="DigNum (strict)"() -> ("Value"=w412:u32)  [unwired: 2 in, 2 out]
                n471 = call "update2dViewer.vi"("nos"=w412, "cam"=u16 0, "cur_nob"=w411) -> ()  [unwired: 8 in, 1 out]
              }
              frame #1 {
                w451 = 3
                # "3 channel per tdc"
                n472 = property on="Signal Board 1 / Cam1" class="WFGraph (strict)"() -> ("Value"=w458:u16[])  [unwired: 2 in, 2 out]
                n473 = Index Array(array=w458, index=7) -> (element=w459:u16)
                n474 = Index Array(array=w458, index=6) -> (element=w461:u16)
                n475 = And(x=w459, y=u16 65535) -> (x .and. y?=w450:u16)
                n476 = And(x=w461, y=u16 65535) -> (x .and. y?=w452:u16)
                n477 = Divide(x=w452, y=w451) -> (x/y=w453:dbl)
                n478 = global read "Globals.vi" "GPX Offset"() -> (w457:u32)
                n479 = Divide(x=w450, y=w451) -> (x/y=w456:dbl)
                n480 = Subtract(x=w453, y=w457) -> (x-y=→"TDC 1":dbl)
                n481 = Subtract(x=w456, y=w457) -> (x-y=→"TDC 2":dbl)
              }
            }
          }
          event "Pixel for Graph": Value Change {
            n482 = event-data() -> ()  [unwired: 1 in, 6 out]
            n483 = property on="no.of blocks (nob)" class="DigNum (strict)"() -> ("Value"=w465:u32)  [unwired: 2 in, 2 out]
            n484 = for {
              N: w465 -> [_]
              tunnel: [w468] -> w466 mode=indexing
              i -> [w469]
              n485 = property on="no.of samples (nos)" class="DigNum (strict)"() -> ("Value"=w467:u32)  [unwired: 2 in, 2 out]
              n486 = for {
                N: w467 -> [_]
                tunnel: w469 -> [w474]
                tunnel: [w473] -> w468 mode=indexing
                i -> [w475]
                n487 = call "ReturnFrame.vi"("curr_nob"=w474, "curr_nos"=w475, "curr_cam"=u16 0) -> ("Data Values Out 1"=w470:u16[])  [unwired: 6 in, 2 out]
                n488 = Index Array(array=w470, index="Pixel for Graph") -> (element=w473:u16)
              }
            }
            "One Pixel Graph" <- w466
          }
          event "About S0": Mouse Down {
            n489 = event-data() -> ()  [unwired: 1 in, 8 out]
            n490 = call "aboutS0.vi"() -> ()  [unwired: 10 in, 1 out]
          }
          event "Reset DSC": Value Change {
            n491 = event-data() -> ()  [unwired: 1 in, 6 out]
            n492 = case shown="True" "Reset DSC" {
              frame False {
              }
              frame True {
                n493 = flat-sequence {
                  frame #0 {
                    w478 = u8 124 items=["S0Addr_CtrlA"=4, "S0Addr_CtrlB"=5, "S0Addr_CtrlC"=6, "S0Addr_XCKLL"=8, "S0Addr_XCKLH"=9, "S0Addr_XCKHL"=10, "S0Addr_XCKMSB"=11, "S0Addr_XCKCNTLL"=12, "S0Addr_XCKCNTLH"=13, "S0Addr_XCKCNTHL"=14, "S0Addr_XCKCNTMSB"=15, "S0Addr_PIXREGlow"=16, "S0Addr_PIXREGhigh"=17, "S0Addr_FREQREG"=18, "S0Addr_FF_FLAGS"=19, "S0Addr_FIFOCNT"=20, "S0Addr_VCLKCTRL"=24, "S0Addr_EBST"=28, "S0Addr_DAT"=32, "S0Addr_EC"=36, "S0Addr_TOR"=40, "S0Addr_ARREG"=44, "S0Addr_GIOREG"=48, "S0Addr_DELAYEC"=52, "S0Addr_IRQREG"=56, "S0Addr_PCI"=60, "R30"=124]
                    n494 = call "WriteL.vi"("val"=u32 1, "offset"=w478) -> ()  [unwired: 9 in, 1 out]
                  }
                  frame #1 {
                    n495 = call "Time Delay"() -> ()  [unwired: 11 in, 1 out]
                  }
                  frame #2 {
                    w480 = u8 124 items=["S0Addr_CtrlA"=4, "S0Addr_CtrlB"=5, "S0Addr_CtrlC"=6, "S0Addr_XCKLL"=8, "S0Addr_XCKLH"=9, "S0Addr_XCKHL"=10, "S0Addr_XCKMSB"=11, "S0Addr_XCKCNTLL"=12, "S0Addr_XCKCNTLH"=13, "S0Addr_XCKCNTHL"=14, "S0Addr_XCKCNTMSB"=15, "S0Addr_PIXREGlow"=16, "S0Addr_PIXREGhigh"=17, "S0Addr_FREQREG"=18, "S0Addr_FF_FLAGS"=19, "S0Addr_FIFOCNT"=20, "S0Addr_VCLKCTRL"=24, "S0Addr_EBST"=28, "S0Addr_DAT"=32, "S0Addr_EC"=36, "S0Addr_TOR"=40, "S0Addr_ARREG"=44, "S0Addr_GIOREG"=48, "S0Addr_DELAYEC"=52, "S0Addr_IRQREG"=56, "S0Addr_PCI"=60, "R14"=120, "R15"=124]
                    n496 = call "WriteL.vi"("val"=u32 0, "offset"=w480) -> ()  [unwired: 9 in, 1 out]
                  }
                }
              }
            }
          }
          event "Read ADSC": Value Change {
            n497 = event-data() -> ()  [unwired: 1 in, 6 out]
            n498 = case shown="True" "Read ADSC" {
              frame False {
              }
              frame True {
                n499 = flat-sequence {
                  frame #0 {
                    w482 = u8 120 items=["S0Addr_CtrlA"=4, "S0Addr_CtrlB"=5, "S0Addr_CtrlC"=6, "S0Addr_XCKLL"=8, "S0Addr_XCKLH"=9, "S0Addr_XCKHL"=10, "S0Addr_XCKMSB"=11, "S0Addr_XCKCNTLL"=12, "S0Addr_XCKCNTLH"=13, "S0Addr_XCKCNTHL"=14, "S0Addr_XCKCNTMSB"=15, "S0Addr_PIXREGlow"=16, "S0Addr_PIXREGhigh"=17, "S0Addr_FREQREG"=18, "S0Addr_FF_FLAGS"=19, "S0Addr_FIFOCNT"=20, "S0Addr_VCLKCTRL"=24, "S0Addr_EBST"=28, "S0Addr_DAT"=32, "S0Addr_EC"=36, "S0Addr_TOR"=40, "S0Addr_ARREG"=44, "S0Addr_GIOREG"=48, "S0Addr_DELAYEC"=52, "S0Addr_IRQREG"=56, "S0Addr_PCI"=60, "R14"=120, "R15"=124]
                    n500 = call "WriteL.vi"("val"=u32 1, "offset"=w482) -> ()  [unwired: 9 in, 1 out]
                  }
                  frame #1 {
                    n501 = call "Time Delay2"() -> ()  [unwired: 11 in, 1 out]
                  }
                  frame #2 {
                    w485 = u8 120 items=["S0Addr_CtrlA"=4, "S0Addr_CtrlB"=5, "S0Addr_CtrlC"=6, "S0Addr_XCKLL"=8, "S0Addr_XCKLH"=9, "S0Addr_XCKHL"=10, "S0Addr_XCKMSB"=11, "S0Addr_XCKCNTLL"=12, "S0Addr_XCKCNTLH"=13, "S0Addr_XCKCNTHL"=14, "S0Addr_XCKCNTMSB"=15, "S0Addr_PIXREGlow"=16, "S0Addr_PIXREGhigh"=17, "S0Addr_FREQREG"=18, "S0Addr_FF_FLAGS"=19, "S0Addr_FIFOCNT"=20, "S0Addr_VCLKCTRL"=24, "S0Addr_EBST"=28, "S0Addr_DAT"=32, "S0Addr_EC"=36, "S0Addr_TOR"=40, "S0Addr_ARREG"=44, "S0Addr_GIOREG"=48, "S0Addr_DELAYEC"=52, "S0Addr_IRQREG"=56, "S0Addr_PCI"=60, "R14"=120, "R15"=124]
                    n502 = call "ReadL.vi"("Offset"=w485) -> ("Data 1"=→"ADSC value":u32)  [unwired: 8 in, 2 out]
                  }
                }
              }
            }
          }
          event "SDAT in 10ns": Value Change {
            # "bit31 must be set for enabling DAT(add 0x80000000) to REG 0x20"
            # "is only valid for external trigger!"
            # "this examples shows how to set the DAT (delay after trigger)"
            n503 = event-data() -> ()  [unwired: 1 in, 6 out]
            n504 = Equal To 0?(x="SDAT in 10ns") -> (x = 0?=w487:bool)
            n505 = case shown="True" w487 {
              tunnel: "SDAT in 10ns" -> [w490 _]
              frame False {
                w488 = u8 32 items=["S0Addr_CtrlA"=4, "S0Addr_CtrlB"=5, "S0Addr_CtrlC"=6, "S0Addr_XCKLL"=8, "S0Addr_XCKLH"=9, "S0Addr_XCKHL"=10, "S0Addr_XCKMSB"=11, "S0Addr_XCKCNTLL"=12, "S0Addr_XCKCNTLH"=13, "S0Addr_XCKCNTHL"=14, "S0Addr_XCKCNTMSB"=15, "S0Addr_PIXREGlow"=16, "S0Addr_PIXREGhigh"=17, "S0Addr_FREQREG"=18, "S0Addr_FF_FLAGS"=19, "S0Addr_FIFOCNT"=20, "S0Addr_VCLKCTRL"=24, "S0Addr_EBST"=28, "S0Addr_DAT"=32, "S0Addr_EC"=36, "S0Addr_TOR"=40, "S0Addr_ARREG"=44, "S0Addr_GIOREG"=48, "S0Addr_DELAYEC"=52, "S0Addr_IRQREG"=56, "S0Addr_PCI"=60]
                n506 = Add(x=u32 2147483648, y=w490) -> (x+y=w489:u32)
                n507 = call "WriteL.vi"("val"=w489, "offset"=w488) -> ()  [unwired: 9 in, 1 out]
              }
              frame True {
                w492 = u8 32 items=["S0Addr_CtrlA"=4, "S0Addr_CtrlB"=5, "S0Addr_CtrlC"=6, "S0Addr_XCKLL"=8, "S0Addr_XCKLH"=9, "S0Addr_XCKHL"=10, "S0Addr_XCKMSB"=11, "S0Addr_XCKCNTLL"=12, "S0Addr_XCKCNTLH"=13, "S0Addr_XCKCNTHL"=14, "S0Addr_XCKCNTMSB"=15, "S0Addr_PIXREGlow"=16, "S0Addr_PIXREGhigh"=17, "S0Addr_FREQREG"=18, "S0Addr_FF_FLAGS"=19, "S0Addr_FIFOCNT"=20, "S0Addr_VCLKCTRL"=24, "S0Addr_EBST"=28, "S0Addr_DAT"=32, "S0Addr_EC"=36, "S0Addr_TOR"=40, "S0Addr_ARREG"=44, "S0Addr_GIOREG"=48, "S0Addr_DELAYEC"=52, "S0Addr_IRQREG"=56, "S0Addr_PCI"=60]
                n508 = call "WriteL.vi"("val"=u32 0, "offset"=w492) -> ()  [unwired: 9 in, 1 out]
              }
            }
          }
          event "no.of samples (nos)", "no.of blocks (nob)", "stime[ms]", "btime[ms]": Value Change {
            w499 = 1.0 ("Scale.Range:Minimum")
            # "calculation of MB RAM an SEC and setting scale max"
            n509 = event-data() -> ()  [unwired: 1 in, 7 out]
            n510 = property on="no.of blocks (nob)" class="DigNum (strict)"() -> ("Value"=w497:u32)  [unwired: 2 in, 2 out]
            n511 = property on="no.of samples (nos)" class="DigNum (strict)"() -> ("Value"=w498:u32)  [unwired: 2 in, 2 out]
            n512 = flat-sequence {
              frame #0 {
                # "TODO: calculate with btime"
                n513 = property on="no.of blocks (nob)" class="DigNum (strict)"() -> ("Value"=w507:u32)  [unwired: 2 in, 2 out]
                n514 = property on="no.of samples (nos)" class="DigNum (strict)"() -> ("Value"=w506:u32)  [unwired: 2 in, 2 out]
                n515 = call "CalcMeasureTimeInSeconds.vi"("exposure_time_in_ms"="stime[ms]", "nob"=w507, "nos"=w506) -> ("measureTimeInSeconds"=→"SEC":dbl)  [unwired: 7 in, 1 out]
              }
              frame #1 {
                n516 = property on="stime[ms]" class="DigNum (strict)"() -> ("Value"=w508:dbl)  [unwired: 2 in, 2 out]
                n517 = global write "Globals.vi" "stime[ms]"(w508) -> ()
                n518 = global write "Globals.vi" "btime[ms]"("btime[ms]") -> ()
              }
              frame #2 {
                n519 = call "SetSTimer.vi"() -> ()  [unwired: 11 in, 1 out]
                n520 = call "SetBTimer.vi"() -> ()  [unwired: 11 in, 1 out]
              }
            }
            n521 = To Double Precision Float(number="no.of samples (nos)") -> (double precision float=w501:dbl)
            n522 = To Double Precision Float(number="no.of blocks (nob)") -> (double precision float=w500:dbl)
            n523 = global write "Globals.vi" "nob"(w497) -> ()
            n524 = global write "Globals.vi" "nos"(w498) -> ()
            n525 = property on="sample" class="Slide (strict)"("Scale.Maximum"=w501) -> ()  [unwired: 2 in, 2 out]
            n526 = property on="block" class="Slide (strict)"("Scale.Maximum"=w500) -> ()  [unwired: 2 in, 2 out]
            n527 = property on="block" class="Slide (strict)"("Maximum"=w500) -> ()  [unwired: 2 in, 2 out]
            n528 = property on="no.of blocks (nob)" class="DigNum (strict)"() -> ("Value"=w494:u32)  [unwired: 2 in, 2 out]
            n529 = property on="sample" class="Slide (strict)"("Maximum"=w501) -> ()  [unwired: 2 in, 2 out]
            n530 = property on="no.of samples (nos)" class="DigNum (strict)"() -> ("Value"=w495:u32)  [unwired: 2 in, 2 out]
            n531 = call "CalcRamUsage.vi"("nob"=w494, "nos"=w495) -> ("ramUsage"=→"MB RAM":dbl)  [unwired: 7 in, 1 out]
            n532 = property on="sample" class="Slide (strict)"("Scale.Minimum"=w499) -> ()  [unwired: 2 in, 2 out]
            n533 = property on="block" class="Slide (strict)"("Scale.Minimum"=w499) -> ()  [unwired: 2 in, 2 out]
            n534 = property on="block" class="Slide (strict)"("Minimum"=w499) -> ()  [unwired: 2 in, 2 out]
            n535 = property on="sample" class="Slide (strict)"("Minimum"=w499) -> ()  [unwired: 2 in, 2 out]
          }
          event "cool": Value Change {
            # "only for cooled cameras"
            # "set cooling level"
            n536 = event-data() -> ()  [unwired: 1 in, 6 out]
            n537 = global read "Globals.vi" "CoolCam"() -> (w510:bool)
            n538 = case shown="True" w510 {
              frame False {
              }
              frame True {
                n539 = flat-sequence {
                  frame #0 {
                    n540 = global write "Globals.vi" "cool level"("cool") -> ()
                  }
                  frame #1 {
                    n541 = call "SetTemp.vi"() -> ()  [unwired: 11 in, 1 out]
                  }
                }
              }
            }
          }
          event "exit": Mouse Down {
            # "exit"
            n542 = event-data() -> ()  [unwired: 1 in, 8 out]
            n543 = stacked-sequence {
              tunnel: [_ TRUE] -> w512
              frame #0 {
                n544 = property on="show greyscale viewer" class="Bool (strict)"("Value"=FALSE) -> ()  [unwired: 2 in, 2 out]
                n545 = call "deinit2dViewer.vi"() -> ()  [unwired: 11 in, 1 out]
              }
              frame #1 {
                # "do not omit, or next call of driver will go wrong."
                n546 = call "Exit.vi"() -> ()  [unwired: 11 in, 1 out]
              }
            }
          }
          event "abort": Mouse Down {
            n547 = event-data() -> ()  [unwired: 1 in, 8 out]
            n548 = dll-call lib="C:/ENTW/PCIE/LV64/board.vis/ESLSCDLL.dll" fn="DLLAbortMeasurement" ("lwlscdll.dll:DLLWriteLongS0")("drvno"=u32 1) -> ()  [unwired: 5 in, 2 out]
          }
          event "TRMS Pix": Value Change {
            w517 = u32 10  # firstSample
            w524 = u32 500
            # "CHA"
            n549 = event-data() -> ()  [unwired: 1 in, 6 out]
            n550 = global read "Globals.vi" "CAMCNT"() -> (w523:u32)
            n551 = property on="no.of samples (nos)" class="DigNum (strict)"() -> ("Value"=w520:u32)  [unwired: 2 in, 2 out]
            n552 = Greater?(x=w520, y=w524) -> (0:w529:bool)
            n553 = Greater?(x=w523, y=u32 1) -> (0:w521:bool)
            n554 = case shown="False" w529 {
              tunnel: [w543 w544] -> w518
              tunnel: w524 -> [_ w544]
              tunnel: w520 -> [w543 _]
              frame False {
              }
              frame True {
              }
            }
            n555 = case shown="True" w521 {
              tunnel: w524 -> [_ w535]
              tunnel: "TRMS Pix" -> [_ w532]
              frame False {
              }
              frame True {
                w530 = u32 10  # firstSample
                # "CHB"
                n556 = property on="no.of samples (nos)" class="DigNum (strict)"() -> ("Value"=w534:u32)  [unwired: 2 in, 2 out]
                n557 = Greater?(x=w534, y=w535) -> (0:w540:bool)
                n558 = case shown="True" w540 {
                  tunnel: [w541 w542] -> w531
                  tunnel: w535 -> [_ w542]
                  tunnel: w534 -> [w541 _]
                  frame False {
                  }
                  frame True {
                  }
                }
                n559 = call "CalcTrms.vi"("CAMpos"=u16 1, "TRMSpix"=w532, "lastSample"=w531, "firstSample"=w530) -> ("TRMS 2"=→"tRMS 3":dbl, "mean 2"=→"mean 3":dbl, "TRMS 1"=→"tRMSB":dbl, "mean 1"=→"meanB":dbl)  [unwired: 3 in, 1 out]
              }
            }
            n560 = call "CalcTrms.vi"("CAMpos"=u16 0, "TRMSpix"="TRMS Pix", "lastSample"=w518, "firstSample"=w517) -> ("TRMS 2"=→"tRMS 2":dbl, "mean 2"=→"mean 2":dbl, "TRMS 1"=→"tRMSA":dbl, "mean 1"=→"meanA":dbl)  [unwired: 3 in, 1 out]
          }
          event "ADC mode", "custom patt: 14bits pattern hex (14bit)": Value Change {
            n561 = event-data() -> ()  [unwired: 1 in, 6 out]
            n562 = case shown="\"2\"" "ADC mode" {
              tunnel: [w548 w549 w550] -> w546
              frame "1" {
                w548 = u8 2  # adc mode
                # "Custom Pattern"
              }
              frame "2" {
                w549 = u8 1  # adc mode
                # "Ramp"
              }
              frame "3" {
                w550 = u8 0  # adc mode
                # "Normal Mode"
              }
            }
            n563 = call "InitCam3030.vi"("custom_pattern"="custom patt: 14bits pattern hex (14bit)", "adc_mode"=w546) -> ()  [unwired: 8 in, 1 out]
            "pattern dec" <- "custom patt: 14bits pattern hex (14bit)"
          }
          event "Offset": Value Change {
            n564 = event-data() -> ()  [unwired: 1 in, 6 out]
            n565 = flat-sequence {
              frame #0 {
                n566 = global read "Globals.vi" "board_sel"() -> (w551:u32)
                n567 = case shown="1" w551 {
                  frame 2 {
                    n568 = property on="Offset" class="Bool (strict)"("Value"=TRUE) -> ()  [unwired: 2 in, 2 out]
                  }
                  frame 3, Default {
                  }
                  frame 1 {
                    n569 = property on="Offset" class="Bool (strict)"("Value"=FALSE) -> ()  [unwired: 2 in, 2 out]
                  }
                }
              }
              frame #1 {
                n570 = case shown="True" "Offset" {
                  tunnel: [FALSE TRUE] -> w555
                  tunnel: [TRUE FALSE] -> w556
                  frame False {
                    n571 = global write "Globals.vi" "board_sel_offset"(u32 1) -> ()
                  }
                  frame True {
                    n572 = global write "Globals.vi" "board_sel_offset"(u32 2) -> ()
                  }
                }
                n573 = global read "Globals.vi" "use DAC"() -> (w554:bool)
                n574 = And(x=w555, y=w554) -> ()  [unwired: 1 out]
                n575 = And(x=w554, y=w556) -> (x .and. y?=w557:bool)
                n576 = property on="DAC 4/ 1" class="DigNum (strict)"("Visible"=w557) -> ()  [unwired: 2 in, 2 out]
                n577 = property on="DAC 2/ 1" class="DigNum (strict)"("Visible"=w557) -> ()  [unwired: 2 in, 2 out]
                n578 = property on="DAC 3/ 1" class="DigNum (strict)"("Visible"=w557) -> ()  [unwired: 2 in, 2 out]
                n579 = property on="DAC 1/ 1" class="DigNum (strict)"("Visible"=w557) -> ()  [unwired: 2 in, 2 out]
                n580 = property on="DAC 5/ 1" class="DigNum (strict)"("Visible"=w557) -> ()  [unwired: 2 in, 2 out]
                n581 = property on="DAC 7/ 1" class="DigNum (strict)"("Visible"=w557) -> ()  [unwired: 2 in, 2 out]
                n582 = property on="DAC 8/ 1" class="DigNum (strict)"("Visible"=w557) -> ()  [unwired: 2 in, 2 out]
                n583 = property on="DAC 6/ 1" class="DigNum (strict)"("Visible"=w557) -> ()  [unwired: 2 in, 2 out]
              }
            }
          }
          event "DAC 2/ 1", "DAC 7/ 1", "DAC 3/ 1", "DAC 8/ 1", "DAC 4/ 1", "DAC 5/ 1", "DAC 1/ 1", "DAC 6/ 1": Value Change {
            w566 = u8 6  # channel
            w568 = u8 3  # channel
            w570 = u8 7  # channel
            w572 = u8 5  # channel
            w574 = u8 1  # channel
            w576 = u8 4  # channel
            w578 = u8 2  # channel
            w580 = u8 0  # channel
            # "CHG"
            # "CHD"
            # "CHH"
            # "CHF"
            # "CHB"
            # "CHE"
            # "CHC"
            # "CHA"
            n584 = event-data() -> ()  [unwired: 1 in, 6 out]
            n585 = call "DAC_setOutput.vi"("output"="DAC 4/ 1", "channel"=w580) -> ()  [unwired: 9 in, 1 out]
            n586 = call "DAC_setOutput.vi"("output"="DAC 5/ 1", "channel"=w574) -> ()  [unwired: 9 in, 1 out]
            n587 = call "DAC_setOutput.vi"("output"="DAC 1/ 1", "channel"=w578) -> ()  [unwired: 9 in, 1 out]
            n588 = call "DAC_setOutput.vi"("output"="DAC 6/ 1", "channel"=w568) -> ()  [unwired: 9 in, 1 out]
            n589 = call "DAC_setOutput.vi"("output"="DAC 8/ 1", "channel"=w570) -> ()  [unwired: 9 in, 1 out]
            n590 = call "DAC_setOutput.vi"("output"="DAC 3/ 1", "channel"=w566) -> ()  [unwired: 9 in, 1 out]
            n591 = call "DAC_setOutput.vi"("output"="DAC 7/ 1", "channel"=w572) -> ()  [unwired: 9 in, 1 out]
            n592 = call "DAC_setOutput.vi"("output"="DAC 2/ 1", "channel"=w576) -> ()  [unwired: 9 in, 1 out]
          }
          event "send all": Value Change {
            n593 = event-data() -> ()  [unwired: 1 in, 6 out]
            n594 = property on="DAC 4/ 1" class="DigNum (strict)"() -> ("Value"=w581:u16)  [unwired: 2 in, 2 out]
            n595 = property on="DAC 4/ 1" class="DigNum (strict)"("Val(Sgnl)"=w581) -> ()  [unwired: 2 in, 2 out]
          }
          event "value white", "value black": Value Change {
            n596 = event-data() -> ()  [unwired: 1 in, 6 out]
            n597 = property on="sample" class="Slide (strict)"() -> ("Value"=w582:u32)  [unwired: 2 in, 2 out]
            n598 = property on="sample" class="Slide (strict)"("Val(Sgnl)"=w582) -> ()  [unwired: 2 in, 2 out]
            n599 = call "setGamma.vi"("black"="value black", "white"="value white") -> ()  [unwired: 10 in]
          }
          event "shutter open": Value Change {
            n600 = event-data() -> ()  [unwired: 1 in, 6 out]
            n601 = case shown="True" "shutter open" {
              frame False {
                # "Close Shutter"
                n602 = call "closeshutter.vi"() -> ()  [unwired: 10 in, 1 out]
              }
              frame True {
                # "Open Shutter"
                n603 = call "OpenShutter.vi"() -> ()  [unwired: 11 in, 1 out]
              }
            }
          }
          event User Event {
            n604 = event-data() -> ()  [unwired: 1 in, 5 out]
            n605 = property on="framewise\ncontinuous" class="Bool (strict)"() -> ("Value"=w588:bool)  [unwired: 2 in, 2 out]
            n606 = property on="fast test\ncontinuous" class="Bool (strict)"() -> ("Value"=w589:bool)  [unwired: 2 in, 2 out]
            n607 = Or(x=w588, y=w589) -> (x .or. y?=w587:bool)
            n608 = case shown="True" w587 {
              frame False {
              }
              frame True {
                n609 = property on="exit" class="Bool (strict)"("DisabledEnum"=2) -> ()  [unwired: 2 in, 2 out]
              }
            }
            "Measure on" <- TRUE
          }
          event User Event {
            # "here could be your math analyses"
            # "Executed after measureOn goes low"
            n610 = event-data() -> ()  [unwired: 1 in, 5 out]
            n611 = disable-structure shown="Disabled" {
              frame Disabled {
                w596 = u32 0  # Block
                w597 = u32 0  # Sample
                w595 = u16 0  # Camera
                # "One specific frame in an 1D array"
                n612 = call "ReturnFrame.vi"("curr_nob"=w596, "curr_nos"=w597, "curr_cam"=w595) -> ()  [unwired: 6 in, 3 out]
              }
              frame Enabled {
              }
            }
            n613 = property on="TRMS Pix" class="DigNum (strict)"() -> ("Value"=w592:u32)  [unwired: 2 in, 2 out]
            n614 = property on="sample" class="Slide (strict)"() -> ("Value"=w593:u32)  [unwired: 2 in, 2 out]
            n615 = disable-structure shown="Disabled" {
              frame Disabled {
                # "All data per PCIe board in an 1D array"
                n616 = call "CopyAllData.vi"() -> ()  [unwired: 9 in, 3 out]
              }
              frame Enabled {
              }
            }
            n617 = property on="Measure on" class="Bool (strict)"("Value"=FALSE) -> ()  [unwired: 2 in, 2 out]
            n618 = property on="TRMS Pix" class="DigNum (strict)"("Val(Sgnl)"=w592) -> ()  [unwired: 2 in, 2 out]
            n619 = property on="sample" class="Slide (strict)"("Val(Sgnl)"=w593) -> ()  [unwired: 2 in, 2 out]
            n620 = property on="exit" class="Bool (strict)"("DisabledEnum"=0) -> ()  [unwired: 2 in, 2 out]
            n621 = flat-sequence {
              frame #0 {
                # "check with scope\nif TOR is set 1"
                # "for test purpose"
                n622 = call "OTrig_h.vi"("drv"=u32 1) -> ()  [unwired: 10 in, 1 out]
              }
              frame #1 {
                n623 = Wait (ms)(milliseconds to wait=10) -> ()  [unwired: 1 out]
              }
              frame #2 {
                n624 = call "OTrig_l.vi"("drv"=u32 1) -> ()  [unwired: 10 in, 1 out]
              }
            }
          }
          event User Event {
            n625 = event-data() -> ()  [unwired: 1 in, 5 out]
            n626 = global read "Globals.vi" "board_sel"() -> (w601:u32)
            n627 = call "ReadB.vi"("Offset"=u32 88) -> ("Data 2"=w602:u8, "Data 1"=w603:u8)  [unwired: 8 in, 1 out]
            n628 = case shown="1, 3, Default" w601 {
              tunnel: [w607 w608] -> w604
              tunnel: w603 -> [_ w608]
              tunnel: w602 -> [w607 _]
              frame 2 {
              }
              frame 1, 3, Default {
              }
            }
            "curr_read_block" <- w604
            "Block on" <- TRUE
          }
          event User Event {
            # "here could be your math analyses"
            # "Executed after one block"
            n629 = event-data() -> ()  [unwired: 1 in, 5 out]
            n630 = disable-structure shown="Disabled" {
              frame Disabled {
                # "Data of the last block in an 1D array"
                n631 = property on="curr_read_block" class="DigNum (strict)"() -> ("Value"=w612:u8)  [unwired: 2 in, 2 out]
                n632 = Subtract(x=w612, y=u8 1) -> (x-y=w611:u8)
                n633 = To Unsigned Word Integer(number=w611) -> (unsigned 16bit integer=w610:u16)
                n634 = call "CopyOneBlock.vi"("block"=w610) -> ()  [unwired: 8 in, 3 out]
              }
              frame Enabled {
              }
            }
            n635 = property on="Block on" class="Bool (strict)"("Value"=FALSE) -> ()  [unwired: 2 in, 2 out]
          }
        }
      }
    }
  }
